vi "Main.vi"(9 "Graph Master":refnum<class "Graph Master.lvclass">=refnum, 10 "MIDA COM":refnum<visa-resource-name>="COM11", 11 "Module Admin":refnum<class "Delacor_lib_QMH_Module Admin.lvclass">) -> ()   [LabVIEW 2023, in "Drive.lvlib"]
doc: "This template is based off of the Queued Message Handler design pattern and the Queued Message Handler project template that ships with LabVIEW.\n\nThe main difference is that the queue is private to this module and communication between modules is performed via Broadcast and Request events.\n\nRequest events are wrapped in public API methods and are handled in the Event Handling Loop (EHL) of this VI. Any module can register for Broadcast events sent by this module. The EHL generates messages based on user interface actions.\n\nThe Message Handling Loop (MHL) processes messages generated by the EHL, or by other messages. The messages are string values, so new messages can be added easily to the Message Cases case structure in the MHL. Each message cluster can also provide an optional value for Message Data, which is a variant that can be converted to whatever message-specific data is required.\n_____\nBased on DQMH Project Template 6.1.0.94."
uses:
  Drive.lvlib
  <vilib>/Delacor/Delacor QMH/Libraries/Message Queue_class/Delacor_lib_QMH_Message Queue.lvclass
  Module Data--cluster.ctl
  <vilib>/Utility/miscctls.llb/LVPointTypeDef.ctl
  <vilib>/Utility/error.llb/Error Cluster From Error Code.vi
  <vilib>/ErrorRing/Error Ring.xnode
  <vilib>/Delacor/Delacor QMH/Libraries/Message Queue_class/Delacor_lib_QMH_Enqueue Message (Single).vi
  Stop Argument--cluster.ctl
  <vilib>/Delacor/Delacor QMH/Libraries/Module Admin_class/Delacor_lib_QMH_Module Admin.lvclass
  Kinco Drive/Kinco Type Class.ctl
  Kinco Drive/Drive_Status Argument--cluster.ctl
  <vilib>/ptbypt/NI_PtbyPt.lvlib
  <vilib>/NI/Modbus Library/API/Wrapper/API Main.lvlib
  <vilib>/NI/Modbus Library/API/Master/Modbus Master.lvclass
  Scheduler/Event Type.ctl
  Scheduler/Stop Argument--cluster.ctl
  Graph_data_collector/Stop event Type.ctl
  Scheduler/Events.ctl
  Scheduler/Init Type.ctl
  Pump_Data_Type.ctl
  Start_Pressure Argument--cluster.ctl
  Start_Mix Argument--cluster.ctl
  Calc_Type.ctl
  <vilib>/Utility/config.llb/NI_LVConfig.lvlib
  PVT_Drive_Type.ctl
  Save Type.ctl
  SubPanel Argument--cluster.ctl
  Rotation Control Type.ctl
  <vilib>/Kortex/Actor Planer/Actor Planer.lvlib
  <vilib>/ActorFramework/Message Enqueuer/Message Enqueuer.lvclass
  Graph Master/rqp_Create Graph.ctl
  KM20 Argument--cluster.ctl
  <vilib>/NI/Modbus Library/API/Wrapper/Create Serial Master.vi
  <vilib>/NI/Modbus Library/API/Wrapper/Create TCP Master.vi
  Mix Type.ctl
  Graph Master/Graph Master.lvclass
panel:
  out "MM PV":dbl(slide) caption="Положение PVT насоса" scale format="%#.2f"
  in  "Pop-Out Tool":bool
  out "P3":dbl caption="Датчик давления Р3" format="%.3f"
  out "P2":dbl caption="Датчик давления Р2" format="%.3f"
  in  "КМ20-40М":bool
  in  "KE":bool
  in  "K 6":bool
  in  "K 5":bool
  in  "K 4":bool
  in  "K 3":bool
  in  "K 2":bool
  in  "K 1":bool
  out "Pressure PV 2":dbl caption="Датчик давления Р4" format="%.3f"
  out "Pressure PV":dbl caption="Датчик давления Р5" format="%.3f"
  in  "TN 2":sgl=12.0 caption="TN" min=0 max=100 format="TN: %#.5f"
  in  "KP 2":sgl=750.0 caption="KP" min=0 max=10000 format="KP: %#.5f"
  in  "Насос":T1={"Mode"=1, "Pressure PV"=0.0, "Pressure SP"=0.0, "Flow PV"=0.0, "Flow SP"=0.0, "Volume PV"=0.0, "Volume SP"=0.0, "MM PV"=0.0, "Start"=FALSE, "Home"=FALSE} {"MM PV" scale format="%#.2f"; "Volume SP" min=0.0 max=1000.0 format="%.3f"; "Volume PV" format="%.3f"; "Flow SP" min=-300.0 max=300.0 format="%.3f"; "Flow PV" format="%.3f"; "Pressure SP" min=0.0 max=99.99 format="%.3f"; "Pressure PV" format="%.3f"; "Mode" items=["Давление"=1, "Расход"=2, "Объём"=3, "Извлечение"=4]}
  in  "Rotate":T2={"Mode"=1, "PV Angle"=0.0, "SP_Angle"=0.0, "Rotate Angle"=0.0, "Timeout"=0.0, "Start"=FALSE, "Home"=FALSE} caption="Поворот" {"Rotate Angle" format="%.1f"; "SP_Angle" format="%.1f"; "PV Angle" format="%.2f"; "Mode" items=["Поворот"=1, "Качание"=2]}
  out "P":dbl format="%.3f МПа"
  in  "TN":sgl=12.0 min=0 max=100 format="TN: %#.5f"
  in  "KP":sgl=750.0 min=0 max=10000 format="KP: %#.5f"
  in  "PVT":T1={"Mode"=1, "Pressure PV"=0.0, "Pressure SP"=0.0, "Flow PV"=0.0, "Flow SP"=0.0, "Volume PV"=0.0, "Volume SP"=0.0, "MM PV"=0.0, "Start"=FALSE, "Home"=FALSE} {"MM PV" scale format="%#.2f"; "Volume SP" min=0.0 max=1000.0 format="%.3f"; "Volume PV" format="%.3f"; "Flow SP" min=-300.0 max=300.0 format="%.3f"; "Flow PV" format="%.3f"; "Pressure SP" min=0.0 max=99.99 format="%.3f"; "Pressure PV" format="%.3f"; "Mode" items=["Давление"=1, "Расход"=2, "Объём"=3, "Извлечение"=4]}
  in  "MIX":T3 caption="Мешалка" {"Q" min=0.0 max=1000.0 format="%#.1f об/мин"}
  out "error out":errorcluster
  # "P2"
  # "P3"
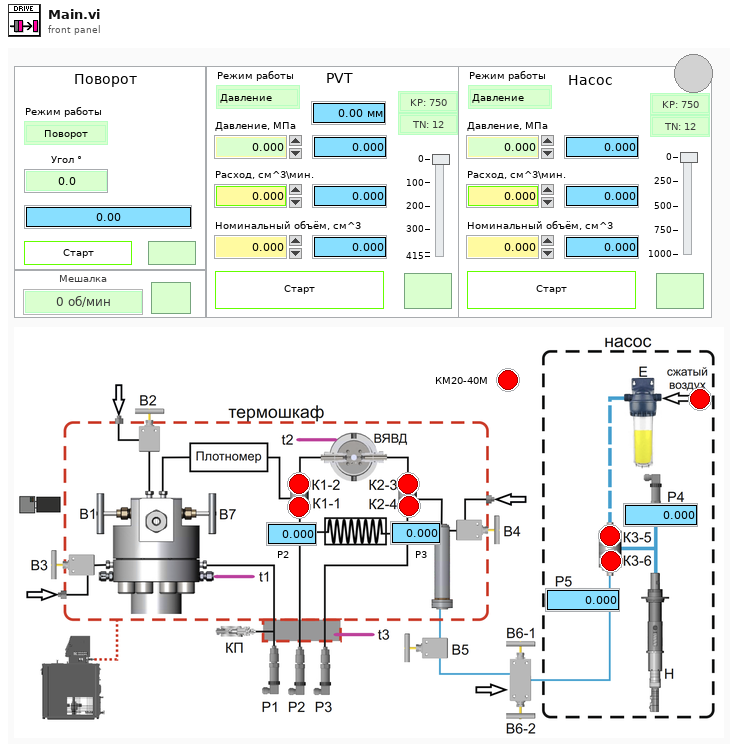
[diagram p1: front panel]
types:
  T1 = typedef "Drive.lvlib/PVT_Drive_Type.ctl" = cluster{"Mode":u16, "Pressure PV":dbl, "Pressure SP":dbl, "Flow PV":dbl, "Flow SP":dbl, "Volume PV":dbl, "Volume SP":dbl, "MM PV":dbl, "Start":bool, "Home":bool}
  T2 = typedef "Drive.lvlib/Rotation Control Type.ctl" = cluster{"Mode":u16, "PV Angle":dbl, "SP_Angle":dbl, "Rotate Angle":dbl, "Timeout":dbl, "Start":bool, "Home":bool}
  T3 = typedef "Drive.lvlib/Mix Type.ctl" = cluster{"Q":dbl, "on":bool}
  T4 = typedef "Kinco Drive.lvlib/Kinco Type Class.ctl" = enum16{"Position", "Speed"}
  T5 = typedef "Drive.lvlib/Request Events--cluster.ctl" = cluster{"Stop Module":refnum<user-event>, "Show Panel":refnum<user-event>, "Hide Panel":refnum<user-event>, "Get Module Execution Status":refnum<user-event>, "Show Diagram":refnum<user-event>, "Start_Pressure":refnum<user-event>, "Start_Mix":refnum<user-event>, "SubPanel":refnum<user-event>, "KM20":refnum<user-event>}
  T6 = typedef "Dispatcher.lvlib/Broadcast Events--cluster.ctl" = cluster{"Module Did Init":refnum<user-event>, "Status Updated":refnum<user-event>, "Error Reported":refnum<user-event>, "Module Did Stop":refnum<user-event>, "Update Module Execution Status":refnum<user-event>, "Emerg Stop Broad":refnum<user-event>}
  T7 = typedef "Settings Master.lvlib/Broadcast Events--cluster.ctl" = cluster{"Module Did Init":refnum<user-event>, "Status Updated":refnum<user-event>, "Error Reported":refnum<user-event>, "Module Did Stop":refnum<user-event>, "Update Module Execution Status":refnum<user-event>, "Settings":refnum<user-event>}
  T8 = typedef "Kinco Drive.lvlib/Broadcast Events--cluster.ctl" = cluster{"Module Did Init":refnum<user-event>, "Status Updated":refnum<user-event>, "Error Reported":refnum<user-event>, "Module Did Stop":refnum<user-event>, "Update Module Execution Status":refnum<user-event>, "Drive_Status":refnum<user-event>}
  T9 = typedef "Heat UI.lvlib/Broadcast Events--cluster.ctl" = cluster{"Module Did Init":refnum<user-event>, "Status Updated":refnum<user-event>, "Error Reported":refnum<user-event>, "Module Did Stop":refnum<user-event>, "Update Module Execution Status":refnum<user-event>, "T Data":refnum<user-event>, "Temp array":refnum<user-event>}
  T10 = typedef "Drive.lvlib/Module Data--cluster.ctl" = cluster{"Status":string, "Mix_ID":i32, "Rotate_ID":i32, "Rotate status":T11, "MB":refnum<class "Modbus Master.lvclass">, "Init":T12, "Temp array":dbl[], "Расчёты":T15, "Plan Enqueuer":refnum<class "Message Enqueuer.lvclass">, "mida":refnum<class "Modbus Master.lvclass">, "Subpanel Ref":refnum<vi>}
  T11 = typedef "Kinco Drive.lvlib/Drive_Status Argument--cluster.ctl" = cluster{"Module ID":i32, "Connection":bool, "is Home?":bool, "Position":dbl, "Done?":bool}
  T12 = typedef "Scheduler Lib.lvlib/Init Type.ctl" = cluster{"Message Queue in":refnum<class "Delacor_lib_QMH_Message Queue.lvclass">, "Events":T13}
  T13 = typedef "Scheduler Lib.lvlib/Events.ctl" = cluster{"Stop Module":T14, "Add event":refnum<user-event>}
  T14 = typedef "Scheduler Lib.lvlib/Stop event Type.ctl" = refnum<user-event>
  T15 = typedef "Drive.lvlib/Calc_Type.ctl" = cluster{"Vm0":dbl, "aa":dbl, "bb":dbl, "K0":dbl, "A":dbl, "B":dbl}
  T16 = enum32{"invalid lock state", "Not Locked", "Locked (No Password)", "Password-protected"}
  T17 = typedef "Drive.lvlib/Stop Argument--cluster.ctl" = cluster{"Origin":string, "Exit via Stop Module Req?":bool, "Wait for Module to stop?":bool}
  T18 = typedef "Graph Master.lvclass/rqp_Create Graph.ctl" = cluster{"Control ref":refnum<vi>}
  T19 = typedef "Drive.lvlib/Start_Pressure Argument--cluster.ctl" = cluster{"Pressure":dbl, "Start":bool}
  T20 = typedef "Drive.lvlib/Start_Mix Argument--cluster.ctl" = cluster{"RPM":dbl, "Start":bool}
  T21 = typedef "Drive.lvlib/SubPanel Argument--cluster.ctl" = cluster{"Sub Panel":refnum<vi>}
  T22 = typedef "Drive.lvlib/KM20 Argument--cluster.ctl" = cluster{"Обдув":bool}
  T23 = typedef "LVPointTypeDef.ctl" = cluster{"Horizontal":i16, "Vertical":i16}
  T24 = enum32{"Invalid", "Standard", "Closed", "Hidden", "Minimized", "Maximized"}
  T25 = typedef "Drive.lvlib/Pump_Data_Type.ctl" = cluster{"Pressure PV":dbl, "Flow PV":dbl, "Volume PV":dbl, "Position_MM":dbl, "Volume corrected":dbl, "mix rpm":dbl}
  T26 = enum8{"Enabled", "Disabled", "Disabled and Grayed Out"}
  T27 = typedef "Drive.lvlib/Save Type.ctl" = cluster{"Q mix":dbl, "Angle":dbl, "KP":sgl, "TN":sgl, "PVT":T1, "Rotate":T2, "Насос":T1, "KP 2":sgl, "TN 2":sgl}
  T28 = typedef "Heat UI.lvlib/Settings Type.ctl" = cluster{"KPтерм":dbl, "TNтерм":dbl, "KPниз":dbl, "TNниз":dbl, "COM ADC":refnum<visa-resource-name>, "COM Termex":refnum<visa-resource-name>, "KPдд":dbl, "TNдд":dbl, "Multiper":dbl}
  T29 = typedef "Menu.lvlib/Setts.ctl" = cluster{"IP adress":string}
  T30 = cluster{"Heat":T28, "Расчёты":T15, "Видеосистема":bool, "Anton Paar":T29, "MIDA COM":refnum<visa-resource-name>}
  T31 = typedef "NI_LVConfig.lvlib/Config Data RefNum.ctl" = refnum<k1>
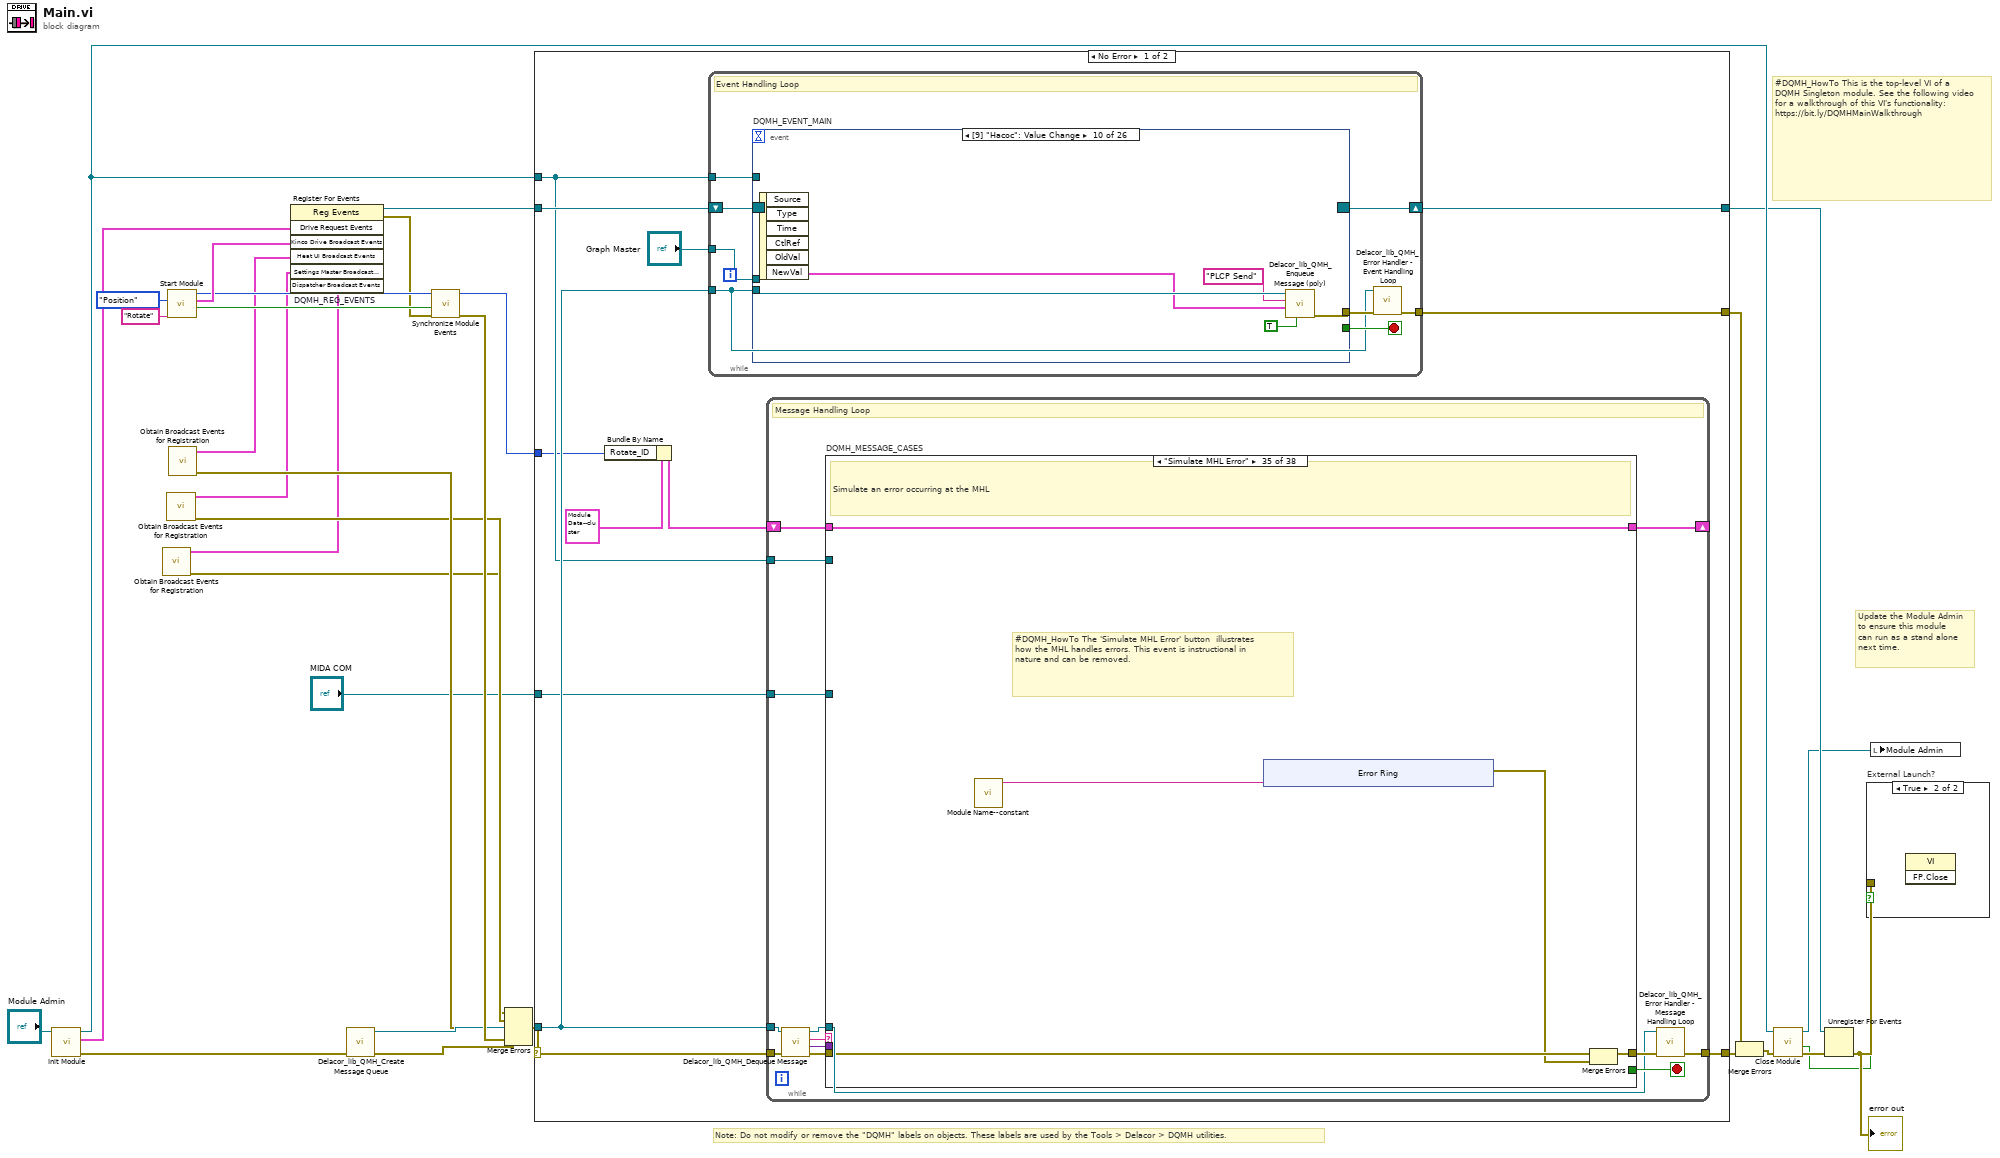
[diagram p0: block diagram]
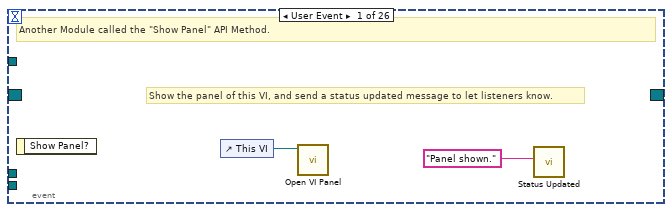
[diagram p3: hidden frame]
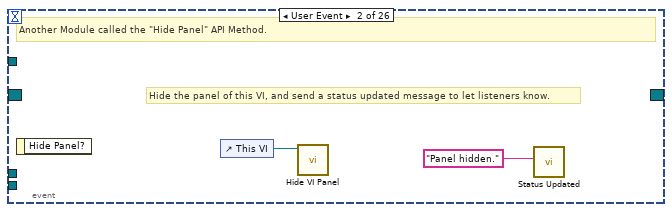
[diagram p4: hidden frame]
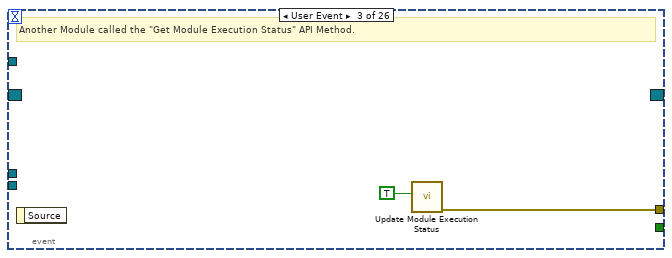
[diagram p5: hidden frame]
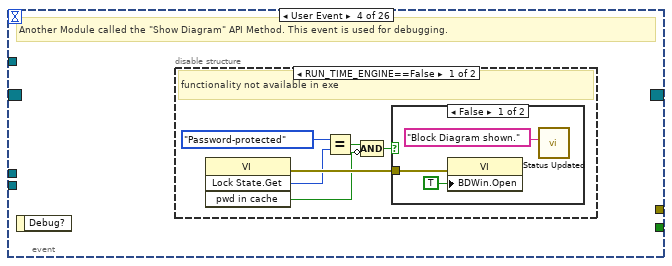
[diagram p6: hidden frame]
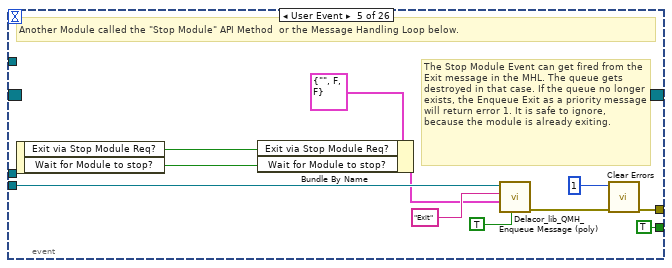
[diagram p9: hidden frame]
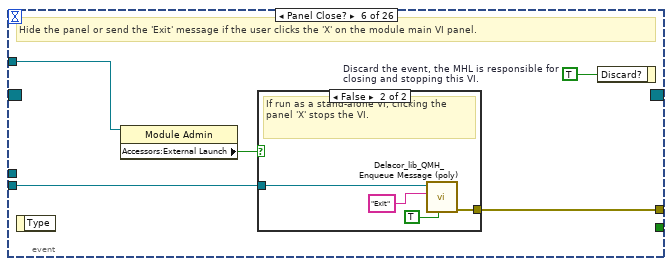
[diagram p10: hidden frame]
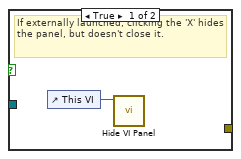
[diagram p11: hidden frame]
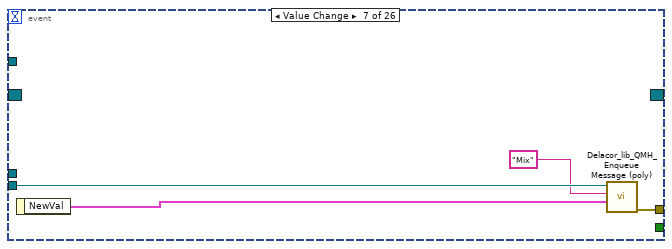
[diagram p12: hidden frame]
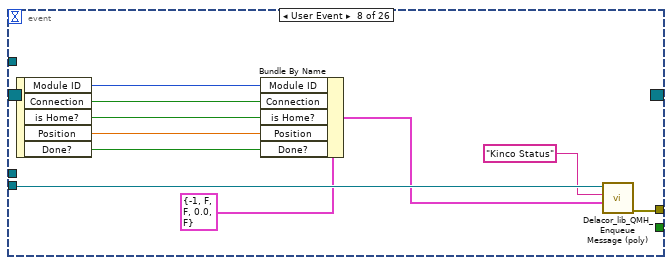
[diagram p13: hidden frame]
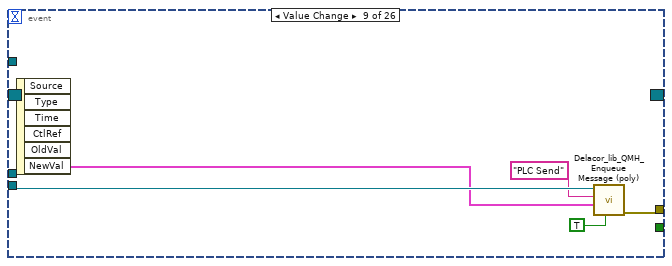
[diagram p14: hidden frame]
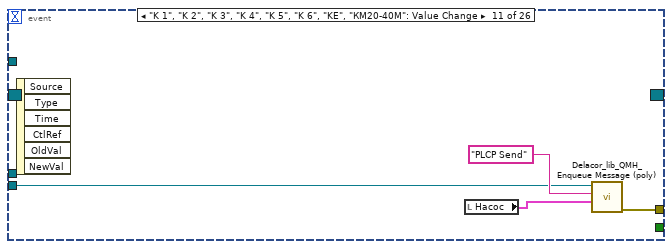
[diagram p15: hidden frame]
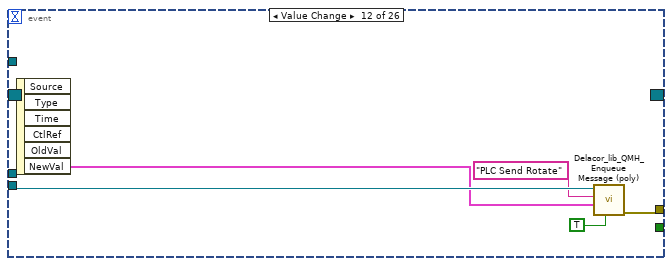
[diagram p16: hidden frame]
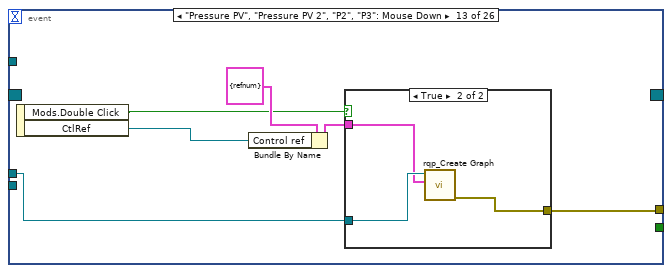
[diagram p17: hidden frame]
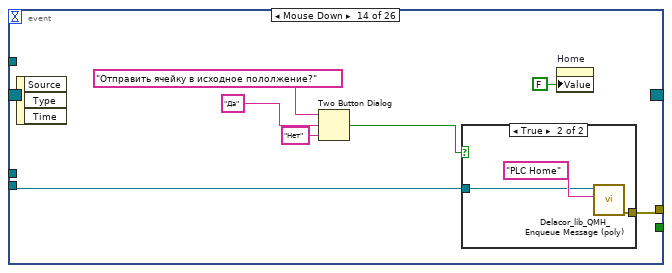
[diagram p19: hidden frame]
diagram:
  # "#DQMH_HowTo This is the top-level VI of a DQMH Singleton module. See the following video for a walkthrough of this VI's functionality: https://bit.ly/DQMHMainWalkthrough"
  # "Note: Do not modify or remove the \"DQMH\" labels on objects. These labels are used by the Tools > Delacor > DQMH utilities."
  # "Update the Module Admin to ensure this module can run as a stand alone next time."
  n1 = call "Init Module.vi"("Singleton Module Admin in"="Module Admin") -> ("error out"=w30:errorcluster, "Drive Request Events"=w8:T5, "Singleton Module Admin out"=w23:refnum<class "Delacor_lib_QMH_Module Admin.lvclass">)  [unwired: 8 in]
  n2 = call "Obtain Broadcast Events for Registration.vi"() -> ("error out"=w2:errorcluster, "Dispatcher Broadcast Events"=w3:T6)  [unwired: 9 in, 1 out]
  n3 = call "Obtain Broadcast Events for Registration.vi"() -> ("error out"=w4:errorcluster, "Settings Master Broadcast Events"=w5:T7)  [unwired: 9 in, 1 out]
  n4 = call "Start Module.vi"("File_name"="Rotate", "Kinco Type"=Kinco_Type_Class."Position") -> ("Wait for Event Sync?"=w16:bool, "Kinco Drive Broadcast Events"=w17:T8, "Module ID"=w15:i32)  [unwired: 6 in, 1 out]
  n5 = call "Obtain Broadcast Events for Registration.vi"() -> ("error out"=w6:errorcluster, "Heat UI Broadcast Events"=w7:T9)  [unwired: 9 in, 1 out]
  n6 = register-events "DQMH_REG_EVENTS"(w8, w17, w7, w5, w3) -> (reference out=w21:refnum<event-registration>, error out=w10:errorcluster)  [unwired: 2 in]
  n7 = call <vilib>:"Delacor_lib_QMH_Create Message Queue.vi"("error in"=w30) -> ("error out"=w25:errorcluster, "Message Queue"=w9:refnum<class "Delacor_lib_QMH_Message Queue.lvclass">)  [unwired: 9 in]
  n8 = call "Synchronize Module Events.vi"("error in"=w10, "Wait for Event Sync?"=w16, "Module ID in"=w15) -> ("error out"=w11:errorcluster, "Module ID out"=w12:i32)  [unwired: 7 in]
  n9 = Merge Errors(w2, w4, w6, w11, w25) -> (w24:errorcluster)
  n10 = case shown="No Error" w24 {
    selector: w24 -> [w41 w926]
    tunnel: [w43 w925] -> w31
    tunnel: [w40 w931] -> w22
    tunnel: w21 -> [w38 w931]
    tunnel: w9 -> [w37 w924]
    tunnel: [w42 _] -> w28
    tunnel: w23 -> [w36 w927]
    tunnel: w12 -> [w34 _]
    tunnel: "MIDA COM" -> [w33 _]
    frame No Error {
      n11 = Bundle By Name(cluster=T10 {"Status"="", "Mix_ID"=0, "Rotate_ID"=0, "Rotate status"={"Module ID"=0, "Connection"=FALSE, "is Home?"=FALSE, "Position"=0.0, "Done?"=FALSE}, "MB"=refnum, "Init"={"Message Queue in"=refnum, "Events"={"Stop Module"=refnum, "Add event"=refnum}}, "Temp array"=[], "Расчёты"={"Vm0"=8.0, "aa"=8.0, "bb"=8.0, "K0"=8.0, "A"=8.0, "B"=8.0}, "Plan Enqueuer"=refnum, "mida"=refnum, "Subpanel Ref"=refnum} ("Data Cluster"), "Rotate_ID"=w34) -> (w35:T10)
      n12 = while {
        tunnel: w37 -> [w45]
        shift-right: [w48] -> w40
        shift-left: w38 -> [w49]
        tunnel: [w50] -> w42
        tunnel: w36 -> [w46]
        tunnel: "Graph Master" -> [w44]
        stop <- w47 stop-if-true
        # "Event Handling Loop"
        n13 = event "DQMH_EVENT_MAIN" shown="[9] \"Насос\": Value Change" {
          selector: w49 -> [_ _ _ _ _ _ _ _ _ _ _ _ _ _ _ _ _ _ _ _ _ _ _ _ _ _]
          dyn-events: [_ _ _ _ _ _ _ _ _ _ _ _ _ _ _ _ _ _ _ _ _ _ _ _ _ _] -> w48
          timeout: _ -> [_ _ _ _ _ _ _ _ _ _ _ _ _ _ _ _ _ _ _ _ _ _ _ _ _ _]
          tunnel: [_ _ _ _ TRUE ("Discard?") _ _ _ _ _ _ _ _ _ _ _ _ _ _ _ _ _ _ _ _ _] -> w47
          tunnel: w45 -> [_ _ _ _ w73 w80 w90 w100 w105 w110 w113 w119 _ w135 w145 w155 w161 w164 w172 w179 w182 w187 w194 _ w205 w206]
          tunnel: [_ _ w57 _ w76 w82 w91 w101 w106 w111 w114 w120 w124 w136 w146 w156 w162 w165 w166 w173 w183 w188 w189 w197 w200 w207] -> w51
          tunnel: w46 -> [_ _ _ _ _ w79 _ _ _ _ _ _ _ _ _ _ _ _ _ _ _ _ _ _ _ _]
          tunnel: w44 -> [_ _ _ _ _ _ _ _ _ _ _ _ w121 _ _ _ _ _ _ _ _ _ _ _ _ _]
          event User Event {
            # "Show the panel of this VI, and send a status updated message to let listeners know."
            # "Another Module called the \"Show Panel\" API Method."
            n14 = event-data() -> ()  [unwired: 1 in, 1 out]
            n15 = control-ref of="This VI"() -> (w53:refnum<vi>)
            n16 = call "Open VI Panel.vi"("VI"=w53) -> ()  [unwired: 10 in, 1 out]
            n17 = call "Status Updated.vi"("Status"="Panel shown." ("format string")) -> ()  [unwired: 10 in, 1 out]
          }
          event User Event {
            # "Hide the panel of this VI, and send a status updated message to let listeners know."
            # "Another Module called the \"Hide Panel\" API Method."
            n18 = event-data() -> ()  [unwired: 1 in, 1 out]
            n19 = control-ref of="This VI"() -> (w55:refnum<vi>)
            n20 = call "Hide VI Panel.vi"("VI"=w55) -> ()  [unwired: 10 in, 1 out]
            n21 = call "Status Updated.vi"("Status"="Panel hidden." ("format string")) -> ()  [unwired: 10 in, 1 out]
          }
          event User Event {
            # "Another Module called the \"Get Module Execution Status\" API Method."
            n22 = event-data() -> ()  [unwired: 1 in, 1 out]
            n23 = call "Update Module Execution Status.vi"("Running?"=TRUE) -> ("error out"=w57:errorcluster)  [unwired: 10 in]
          }
          event User Event {
            # "Another Module called the \"Show Diagram\" API Method. This event is used for debugging."
            n24 = event-data() -> ()  [unwired: 1 in, 1 out]
            n25 = disable-structure shown="RUN_TIME_ENGINE==False" {
              frame condition #0 (active) {
                # "functionality not available in exe"
                n26 = invoke class="VI" method="Lock State.Get"() -> (error out=w63:errorcluster, "Get Lock State"=w62:T16, "pwd in cache"=w59:bool)  [unwired: 4 in, 1 out]
                n27 = Equal?(x=T16."Password-protected", y=w62) -> (x = y?=w60:bool)
                n28 = Compound Arithmetic op=AND(w60, invert w59) -> (w58:bool)
                n29 = case shown="False" w58 {
                  tunnel: w63 -> [w66 _]
                  frame False {
                    n30 = property class="VI"(error in=w66, "BDWin.Open"=TRUE ("Block Diagram Window:Open")) -> ()  [unwired: 1 in, 2 out]
                    n31 = call "Status Updated.vi"("Status"="Block Diagram shown." ("format string")) -> ()  [unwired: 10 in, 1 out]
                  }
                  frame True {
                    # "Password-protected VI, and the password is not in the cache. Do not show the diagram."
                  }
                }
              }
              frame condition #1 {
              }
            }
          }
          event User Event {
            # "The Stop Module Event can get fired from the Exit message in the MHL. The queue gets destroyed in that case. If the queue no longer exists, the Enqueue Exit as a priority message will return error 1. It is safe to ignore, because the module is already exiting."
            # "Another Module called the \"Stop Module\" API Method  or the Message Handling Loop below."
            n32 = event-data() -> ("Exit via Stop Module Req?"=w69:bool, "Wait for Module to stop?"=w68:bool)  [unwired: 1 in]
            n33 = Bundle By Name(cluster=T17 {"Origin"="", "Exit via Stop Module Req?"=FALSE, "Wait for Module to stop?"=FALSE} ("Stop Argument"), "Exit via Stop Module Req?"=w69, "Wait for Module to stop?"=w68) -> (w67:T17)
            n34 = call-poly <vilib>:"Delacor_lib_QMH_Enqueue Message (poly).vi"("Priority Message? (F)"=TRUE, "Message Data"=w67, "Message"="Exit", "Message Queue in"=w73) -> ("error out"=w77:errorcluster)  [unwired: 6 in, 1 out]
            n35 = call <vilib>:"Clear Errors.vi"("error in (no error)"=w77, "specific error code to clear (0: all)"=1) -> ("error out"=w76:errorcluster)  [unwired: 4 in, 1 out]
          }
          event Panel Close? {
            w81 = TRUE  # Discard the event, the MHL is responsible for closing and stopping this VI.
            # "Hide the panel or send the 'Exit' message if the user clicks the 'X' on the module main VI panel."
            n36 = event-data() -> ()  [unwired: 1 in, 1 out]
            n37 = property class="Module Admin"(reference=w79) -> ("Accessors:External Launch"=w78:bool)  [unwired: 1 in, 2 out]
            n38 = case shown="False" w78 {
              tunnel: w80 -> [_ w86]
              tunnel: [_ w87] -> w82
              frame True {
                # "If externally launched, clicking the 'X' hides the panel, but doesn't close it."
                n39 = control-ref of="This VI"() -> (w83:refnum<vi>)
                n40 = call "Hide VI Panel.vi"("VI"=w83) -> ()  [unwired: 10 in, 1 out]
              }
              frame False {
                # "If run as a stand-alone VI, clicking the panel 'X' stops the VI."
                n41 = call-poly <vilib>:"Delacor_lib_QMH_Enqueue Message (poly).vi"("Priority Message? (F)"=TRUE, "Message"="Exit", "Message Queue in"=w86) -> ("error out"=w87:errorcluster)  [unwired: 7 in, 1 out]
              }
            }
            n42 = event-data("Discard?"=w81) -> ()  [unwired: 1 in, 1 out]
          }
          event Value Change {
            n43 = event-data() -> ("NewVal"=w89:T3)  [unwired: 1 in]
            n44 = call-poly <vilib>:"Delacor_lib_QMH_Enqueue Message (poly).vi"("Message Data"=w89, "Message"="Mix", "Message Queue in"=w90) -> ("error out"=w91:errorcluster)  [unwired: 7 in, 1 out]
          }
          event User Event {
            n45 = event-data() -> ("Module ID"=w92:i32, "Connection"=w93:bool, "is Home?"=w94:bool, "Position"=w95:dbl, "Done?"=w96:bool)  [unwired: 1 in]
            n46 = Bundle By Name(cluster=T11 {"Module ID"=-1, "Connection"=FALSE, "is Home?"=FALSE, "Position"=0.0, "Done?"=FALSE} ("Drive_Status Argument"), "Module ID"=w92, "Connection"=w93, "is Home?"=w94, "Position"=w95, "Done?"=w96) -> (w97:T11)
            n47 = call-poly <vilib>:"Delacor_lib_QMH_Enqueue Message (poly).vi"("Message Data"=w97, "Message"="Kinco Status", "Message Queue in"=w100) -> ("error out"=w101:errorcluster)  [unwired: 7 in, 1 out]
          }
          event Value Change {
            n48 = event-data() -> ("NewVal"=w104:T1)  [unwired: 1 in, 5 out]
            n49 = call-poly <vilib>:"Delacor_lib_QMH_Enqueue Message (poly).vi"("Priority Message? (F)"=TRUE, "Message Data"=w104, "Message"="PLC Send", "Message Queue in"=w105) -> ("error out"=w106:errorcluster)  [unwired: 6 in, 1 out]
          }
          event Value Change {
            n50 = event-data() -> ("NewVal"=w109:T1)  [unwired: 1 in, 5 out]
            n51 = call-poly <vilib>:"Delacor_lib_QMH_Enqueue Message (poly).vi"("Priority Message? (F)"=TRUE, "Message Data"=w109, "Message"="PLCP Send", "Message Queue in"=w110) -> ("error out"=w111:errorcluster)  [unwired: 6 in, 1 out]
          }
          event "K 1", "K 2", "K 3", "K 4", "K 5", "K 6", "KE", "КМ20-40М": Value Change {
            n52 = event-data() -> ()  [unwired: 1 in, 6 out]
            n53 = local read "Насос"() -> (w112:T1)
            n54 = call-poly <vilib>:"Delacor_lib_QMH_Enqueue Message (poly).vi"("Message Data"=w112, "Message"="PLCP Send", "Message Queue in"=w113) -> ("error out"=w114:errorcluster)  [unwired: 7 in, 1 out]
          }
          event Value Change {
            n55 = event-data() -> ("NewVal"=w118:T2)  [unwired: 1 in, 5 out]
            n56 = call-poly <vilib>:"Delacor_lib_QMH_Enqueue Message (poly).vi"("Priority Message? (F)"=TRUE, "Message Data"=w118, "Message"="PLC Send Rotate", "Message Queue in"=w119) -> ("error out"=w120:errorcluster)  [unwired: 6 in, 1 out]
          }
          event "Pressure PV", "Pressure PV 2", "P2", "P3": Mouse Down {
            n57 = event-data() -> ("Mods.Double Click"=w123:bool, "CtlRef"=w122:refnum<vi>)  [unwired: 1 in]
            n58 = Bundle By Name(cluster=T18 {"Control ref"=refnum} ("Data in"), "Control ref"=w122) -> (w125:T18)
            n59 = case shown="True" w123 {
              tunnel: w121 -> [_ w129]
              tunnel: [_ w128] -> w124
              tunnel: w125 -> [_ w127]
              frame False {
              }
              frame True {
                n60 = call "rqp_Create Graph.vi"("Data in"=w127, "Graph Master in"=w129) -> ("error out"=w128:errorcluster)  [unwired: 7 in, 2 out]
              }
            }
          }
          event Mouse Down {
            n61 = event-data() -> ()  [unwired: 1 in, 3 out]
            n62 = Two Button Dialog(message="Отправить ячейку в исходное пололжение?", 1:"Нет" ("F button name (\"Cancel\")"), 2:"Да" ("T button name (\"OK\")")) -> (T button?=w130:bool)
            n63 = case shown="True" w130 {
              tunnel: [_ w139] -> w136
              tunnel: w135 -> [_ w137]
              frame False {
              }
              frame True {
                n64 = call-poly <vilib>:"Delacor_lib_QMH_Enqueue Message (poly).vi"("Message"="PLC Home", "Message Queue in"=w137) -> ("error out"=w139:errorcluster)  [unwired: 8 in, 1 out]
              }
            }
            n65 = property on="Home" class="Bool (strict)"("Value"=FALSE) -> ()  [unwired: 2 in, 2 out]
          }
          event Mouse Down {
            n66 = event-data() -> ()  [unwired: 1 in, 3 out]
            n67 = Two Button Dialog(message="Повернуть насос в исходное пололжение?", 1:"Нет" ("F button name (\"Cancel\")"), 2:"Да" ("T button name (\"OK\")")) -> (T button?=w140:bool)
            n68 = case shown="True" w140 {
              tunnel: [_ w149] -> w146
              tunnel: w145 -> [_ w147]
              frame False {
              }
              frame True {
                n69 = call-poly <vilib>:"Delacor_lib_QMH_Enqueue Message (poly).vi"("Message"="PLCP Home", "Message Queue in"=w147) -> ("error out"=w149:errorcluster)  [unwired: 8 in, 1 out]
              }
            }
            n70 = property on="Home" class="Bool (strict)"("Value"=FALSE) -> ()  [unwired: 2 in, 2 out]
          }
          event Mouse Down {
            n71 = event-data() -> ()  [unwired: 1 in, 3 out]
            n72 = Two Button Dialog(message="Повернуть ячейку в исходное пололжение?", 1:"Нет" ("F button name (\"Cancel\")"), 2:"Да" ("T button name (\"OK\")")) -> (T button?=w153:bool)
            n73 = case shown="True" w153 {
              tunnel: [_ w159] -> w156
              tunnel: w155 -> [_ w157]
              frame False {
              }
              frame True {
                n74 = call-poly <vilib>:"Delacor_lib_QMH_Enqueue Message (poly).vi"("Message"="PLC Rotate Home", "Message Queue in"=w157) -> ("error out"=w159:errorcluster)  [unwired: 8 in, 1 out]
              }
            }
            n75 = property on="Home" class="Bool (strict)"("Value"=FALSE) -> ()  [unwired: 2 in, 2 out]
          }
          event "KP", "TN": Value Change {
            n76 = event-data() -> ()  [unwired: 1 in, 6 out]
            n77 = call-poly <vilib>:"Delacor_lib_QMH_Enqueue Message (poly).vi"("Message"="Write PID", "Message Queue in"=w161) -> ("error out"=w162:errorcluster)  [unwired: 8 in, 1 out]
          }
          event "KP 2", "TN 2": Value Change {
            n78 = event-data() -> ()  [unwired: 1 in, 6 out]
            n79 = call-poly <vilib>:"Delacor_lib_QMH_Enqueue Message (poly).vi"("Message"="Write PIDP", "Message Queue in"=w164) -> ("error out"=w165:errorcluster)  [unwired: 8 in, 1 out]
          }
          event User Event {
            # "Another Module called the \"Start_Pressure\" API Method."
            n80 = event-data() -> ("Pressure"=w168:dbl, "Start"=w167:bool)  [unwired: 1 in]
            n81 = Bundle(cluster=T19 {"Pressure"=0.0, "Start"=FALSE} ("Start_Pressure Argument"), "Pressure"=w168, "Start"=w167) -> (w169:T19)
            n82 = call-poly <vilib>:"Delacor_lib_QMH_Enqueue Message (poly).vi"("Message Data"=w169, "Message"="Start_Pressure", "Message Queue in"=w172) -> ("error out"=w166:errorcluster)  [unwired: 7 in, 1 out]
          }
          event User Event {
            # "Another Module called the \"Start_Mix\" API Method."
            n83 = event-data() -> ("RPM"=w175:dbl, "Start"=w174:bool)  [unwired: 1 in]
            n84 = Bundle(cluster=T20 {"RPM"=0.0, "Start"=FALSE} ("Start_Mix Argument"), "RPM"=w175, "Start"=w174) -> (w176:T20)
            n85 = call-poly <vilib>:"Delacor_lib_QMH_Enqueue Message (poly).vi"("Message Data"=w176, "Message"="Start_Mix", "Message Queue in"=w179) -> ("error out"=w173:errorcluster)  [unwired: 7 in, 1 out]
          }
          event User Event {
            n86 = event-data() -> ("Temp array"=w181:dbl[])  [unwired: 1 in]
            n87 = call-poly <vilib>:"Delacor_lib_QMH_Enqueue Message (poly).vi"("Message Data"=w181, "Message"="Temp Data", "Message Queue in"=w182) -> ("error out"=w183:errorcluster)  [unwired: 7 in, 1 out]
          }
          event User Event {
            n88 = event-data() -> ("Main"=w186:T30)  [unwired: 1 in]
            n89 = Unbundle By Name(w186) -> ("Расчёты"=w185:T15)
            n90 = call-poly <vilib>:"Delacor_lib_QMH_Enqueue Message (poly).vi"("Message Data"=w185, "Message"="Setts", "Message Queue in"=w187) -> ("error out"=w188:errorcluster)  [unwired: 7 in, 1 out]
          }
          event User Event {
            # "Another Module called the \"SubPanel\" API Method."
            n91 = event-data() -> ("Sub Panel"=w190:refnum<vi>)  [unwired: 1 in]
            n92 = Bundle(cluster=T21 {"Sub Panel"=refnum} ("SubPanel Argument"), "Sub Panel"=w190) -> (w191:T21)
            n93 = call-poly <vilib>:"Delacor_lib_QMH_Enqueue Message (poly).vi"("Message Data"=w191, "Message"="SubPanel", "Message Queue in"=w194) -> ("error out"=w189:errorcluster)  [unwired: 7 in, 1 out]
          }
          event User Event {
            w196 = FALSE ("Value (Signaling)")
            n94 = event-data() -> ()  [unwired: 1 in, 1 out]
            n95 = property on="Start" class="Bool (strict)"("Val(Sgnl)"=w196) -> (error out=w199:errorcluster)  [unwired: 2 in, 1 out]
            n96 = property on="on" class="Bool (strict)"("Val(Sgnl)"=w196) -> (error out=w198:errorcluster)  [unwired: 2 in, 1 out]
            n97 = property on="Start" class="Bool (strict)"("Val(Sgnl)"=w196) -> (error out=w195:errorcluster)  [unwired: 2 in, 1 out]
            n98 = Merge Errors(w195, w198, w199) -> (w197:errorcluster)
          }
          event User Event {
            # "Another Module called the \"KM20\" API Method."
            n99 = event-data() -> ("Обдув"=w201:bool)  [unwired: 1 in]
            n100 = Bundle(cluster=T22 {"Обдув"=FALSE} ("KM20 Argument"), "Обдув"=w201) -> (w202:T22)
            n101 = call-poly <vilib>:"Delacor_lib_QMH_Enqueue Message (poly).vi"("Message Data"=w202, "Message"="KM20", "Message Queue in"=w205) -> ("error out"=w200:errorcluster)  [unwired: 7 in, 1 out]
          }
          event "Pop-Out Tool": Value Change {
            n102 = event-data() -> ()  [unwired: 1 in, 1 out]
            n103 = call-poly <vilib>:"Delacor_lib_QMH_Enqueue Message (poly).vi"("Message"="Window", "Message Queue in"=w206) -> ("error out"=w207:errorcluster)  [unwired: 8 in, 1 out]
          }
        }
        n104 = call-dynamic "Delacor_lib_QMH_Error Handler - Event Handling Loop.vi"("error in"=w51, "Message Queue in"=w45) -> ("dup error in"=w50:errorcluster)  [unwired: 8 in, 1 out]
      }
      n105 = while {
        tunnel: w37 -> [w212]
        shift-right: [w216] -> _
        shift-left: w35 -> [w217]
        tunnel: w41 -> [w220]
        tunnel: [w218] -> w43
        tunnel: w36 -> [w210]
        tunnel: w33 -> [w209]
        stop <- w215 stop-if-true
        # "Message Handling Loop"
        n106 = call-dynamic "Delacor_lib_QMH_Dequeue Message.vi"("error in"=w220, "Message Queue in"=w212) -> ("error out"=w219:errorcluster, "Message Data"=w213:variant, "Message"=w214:string, "Message Queue out"=w211:refnum<class "Delacor_lib_QMH_Message Queue.lvclass">)  [unwired: 6 in]
        n107 = case "DQMH_MESSAGE_CASES" shown="\"Simulate MHL Error\"" w214 {
          selector: w214 -> [_ _ _ _ _ _ _ _ _ _ _ _ _ _ _ _ _ _ _ _ _ _ _ _ _ _ _ _ _ _ _ _ _ _ _ _ _ w911]
          tunnel: w211 -> [w227 _ _ _ _ _ _ _ _ _ _ w378 _ _ _ _ w475 _ _ _ w540 w604 w640 _ w682 w713 w740 _ _ _ _ _ w810 _ _ w853 w903 _]
          tunnel: w219 -> [w253 w256 w269 w281 w292 w301 w304 w313 w334 w361 w377 w386 w395 w407 w433 w455 w493 w506 _ w528 w557 w614 w651 w678 w694 w724 w744 _ _ w777 w798 w806 w821 w838 w843 w860 w909 w913]
          tunnel: [w236 w256 w258 w271 w286 w294 w303 w312 w333 w360 w376 w385 w394 w409 w435 w457 w492 w508 w522 w530 w556 w613 w650 w679 w695 w725 w745 w759 w773 w783 w803 w808 w822 w838 w842 w856 w906 w914] -> w221
          tunnel: w217 -> [w244 w255 w268 w280 w291 w300 w302 w311 w332 w359 w367 w384 w391 w408 w434 w456 w491 w507 w521 w529 w532 w605 w644 w670 w690 w721 w734 w758 w772 w782 w802 w807 w818 w837 w840 w855 w890 w912]
          tunnel: [w243 w255 w268 w280 w283 w300 w302 w311 w327 w344 w370 w384 w391 w408 w434 w456 w491 w503 w520 w524 w539 w603 w647 w670 w685 w716 w734 w754 w768 w779 w800 w807 w816 w837 w840 w855 w890 w912] -> w216
          tunnel: [_ _ _ _ _ _ _ _ _ _ _ _ _ _ _ _ _ _ _ _ _ _ _ _ _ _ _ _ _ _ _ _ _ _ _ _ w902 _] -> w215
          tunnel: w213 -> [_ _ w266 w278 w289 w298 _ _ _ _ _ _ _ w405 w431 w453 _ w505 _ w527 _ _ _ w677 w693 w723 w743 _ _ _ _ _ w820 _ _ w854 w901 _]
          tunnel: w210 -> [w245 _ _ _ _ _ _ _ _ _ _ _ _ _ _ _ _ _ _ _ _ _ _ _ _ _ _ _ _ _ _ _ _ _ _ w852 w896 _]
          tunnel: w209 -> [_ _ _ _ _ _ _ _ _ _ w362 _ _ _ _ _ _ _ _ _ _ _ _ _ _ _ _ _ _ _ _ _ _ _ _ _ _ _]
          frame "Initialize" {
            # "Initialize - Any operation that needs to be done before the module can receive messages. Synchronize Caller Events.vi will inform Start Module.vi that the module has launched and is ready to receive messages. Module Did Init.vi will broadcast that the module initialized."
            n108 = call "Synchronize Caller Events.vi"("error in (no error)"=w253, "Singleton Module Admin in"=w245) -> ("error out"=w252:errorcluster, "Singleton Module Admin out"=w240:refnum<class "Delacor_lib_QMH_Module Admin.lvclass">)  [unwired: 8 in]
            n109 = property class="Module Admin"(reference=w240) -> ("Accessors:External Launch"=w249:bool)  [unwired: 1 in, 2 out]
            n110 = property on="Pane" class="Pane"("Origin"=T23 {"Horizontal"=0, "Vertical"=0}) -> ()  [unwired: 2 in, 2 out]
            n111 = call-poly <vilib>:"Delacor_lib_QMH_Enqueue Message (poly).vi"("Message"="Load param", "Message Queue in"=w227) -> ("error out"=w230:errorcluster, "Message Queue out"=w228:refnum<class "Delacor_lib_QMH_Message Queue.lvclass">)  [unwired: 8 in]
            n112 = Select(t=T24."Hidden" ("State"), s=w249, f=T24."Standard" ("State")) -> (s? t:f=w246:T24)
            n113 = call-poly <vilib>:"Delacor_lib_QMH_Enqueue Message (poly).vi"("error in"=w230, "Message"="PLC Connect", "Message Queue in"=w228) -> ("error out"=w229:errorcluster, "Message Queue out"=w235:refnum<class "Delacor_lib_QMH_Message Queue.lvclass">)  [unwired: 7 in]
            n114 = call-poly <vilib>:"Delacor_lib_QMH_Enqueue Message (poly).vi"("error in"=w229, "Message"="Read Setts", "Message Queue in"=w235) -> ("error out"=w225:errorcluster, "Message Queue out"=w226:refnum<class "Delacor_lib_QMH_Message Queue.lvclass">)  [unwired: 7 in]
            n115 = call-poly <vilib>:"Delacor_lib_QMH_Enqueue Message (poly).vi"("error in"=w225, "Message"="MIDA open", "Message Queue in"=w226) -> ("error out"=w223:errorcluster, "Message Queue out"=w224:refnum<class "Delacor_lib_QMH_Message Queue.lvclass">)  [unwired: 7 in]
            n116 = call <vilib>:"Start.vi"("DQMH Queue"=w224) -> ("error out"=w231:errorcluster, "Plan Enqueuer"=w232:refnum<class "Message Enqueuer.lvclass">)  [unwired: 9 in]
            n117 = property class="VI"("Front Panel.Title"="Управление движениями" ("Front Panel Window:Title")) -> (reference out=w250:refnum<vi>, error out=w254:errorcluster)  [unwired: 2 in]
            n118 = call "Module Name--constant.vi"() -> ("Module Name"=w241:string)  [unwired: 11 in]
            n119 = invoke class="VI" method="FP.Open"(reference=w250, error in=w254, "State"=w246) -> ()  [unwired: 2 in, 5 out]
            n120 = Bundle By Name(cluster=w244, "Plan Enqueuer"=w232) -> (w243:T10)
            n121 = call "Module Did Init.vi"("error in (no error)"=w252, "Initialized?"=TRUE, "Origin"=w241) -> ("error out"=w251:errorcluster)  [unwired: 8 in]
            n122 = Merge Errors(w231, w223, w251) -> (w236:errorcluster)
          }
          frame "---Module Specific---" {
            # "Separator -- The following cases handle messages specific to this Module."
          }
          frame "Start_Pressure" {
            n123 = Variant To Data(error in=w269, type=T19 {"Pressure"=0.0, "Start"=FALSE} ("Start_Pressure Argument"), Variant=w266) -> (data=w264:T19, error out=w267:errorcluster)
            n124 = Unbundle By Name(w264) -> ("Pressure"=w261:dbl, "Start"=w260:bool)
            n125 = local read "PVT"() -> (w263:T1)
            n126 = Bundle By Name(cluster=w263, "Mode"=u16 1, "Pressure SP"=w261, "Start"=w260) -> (w259:T1)
            n127 = property on="PVT" class="Clust (strict)"("Val(Sgnl)"=w259) -> (error out=w257:errorcluster)  [unwired: 2 in, 1 out]
            n128 = Merge Errors(w257, w267) -> (w258:errorcluster)
          }
          frame "Start_Mix" {
            n129 = Variant To Data(error in=w281, type=T20 {"RPM"=0.0, "Start"=FALSE} ("Start_Mix Argument"), Variant=w278) -> (data=w276:T20, error out=w279:errorcluster)
            n130 = Unbundle By Name(w276) -> ("RPM"=w274:dbl, "Start"=w273:bool)
            n131 = local read "MIX"() -> (w275:T3)
            n132 = Bundle By Name(cluster=w275, "Q"=w274, "on"=w273) -> (w272:T3)
            n133 = property on="MIX" class="Clust (strict)"("Val(Sgnl)"=w272) -> (error out=w270:errorcluster)  [unwired: 2 in, 1 out]
            n134 = Merge Errors(w270, w279) -> (w271:errorcluster)
          }
          frame "SubPanel" {
            n135 = Variant To Data(error in=w292, type=T21 {"Sub Panel"=refnum} ("SubPanel Argument"), Variant=w289) -> (data=w287:T21, error out=w290:errorcluster)
            n136 = Unbundle By Name(w287) -> ("Sub Panel"=w282:refnum<vi>)
            n137 = control-ref of="This VI"() -> (w284:refnum<vi>)
            n138 = Bundle By Name(cluster=w291, "Subpanel Ref"=w282) -> (w283:T10)
            n139 = call "Insert SubPanel.vi"("VI Ref"=w284, "Subpanel Ref"=w282) -> ("error out"=w285:errorcluster)  [unwired: 9 in]
            n140 = Merge Errors(w285, w290) -> (w286:errorcluster)
          }
          frame "KM20" {
            n141 = Variant To Data(error in=w301, type=T22 {"Обдув"=FALSE} ("KM20 Argument"), Variant=w298) -> (data=w296:T22, error out=w299:errorcluster)
            n142 = Unbundle By Name(w296) -> ("Обдув"=w295:bool)
            n143 = property on="КМ20-40М" class="Bool (strict)"("Val(Sgnl)"=w295) -> (error out=w293:errorcluster)  [unwired: 2 in, 1 out]
            n144 = Merge Errors(w293, w299) -> (w294:errorcluster)
          }
          frame "---Copy This Frame---" {
            # "Duplicate this frame when creating new messages.  Change this comment in the duplicated frame to describe this message."
            n145 = Merge Errors(w304) -> (w303:errorcluster)
          }
          frame "Window" {
            # "Duplicate this frame when creating new messages.  Change this comment in the duplicated frame to describe this message."
            n146 = Unbundle By Name(w311) -> ("Subpanel Ref"=w306:refnum<vi>)
            n147 = control-ref of="This VI"() -> (w309:refnum<vi>)
            n148 = invoke class="SubPnl" method="Remove VI"(reference=w306) -> (error out=w307:errorcluster)  [unwired: 2 in, 2 out]
            n149 = invoke class="VI" method="FP.Close"(reference=w309, error in=w307) -> (reference out=w310:refnum<vi>)  [unwired: 1 in, 2 out]
            n150 = invoke class="VI" method="FP.Open"(reference=w310, "State"=T24."Standard") -> (error out=w305:errorcluster)  [unwired: 3 in, 4 out]
            n151 = Merge Errors(w305, w313) -> (w312:errorcluster)
          }
          frame "ReadDO" {
            # "Duplicate this frame when creating new messages.  Change this comment in the duplicated frame to describe this message."
            n152 = Unbundle By Name(w332) -> ("MB"=w331:refnum<class "Modbus Master.lvclass">)
            n153 = call-dynamic "Read Holding Registers.vi"("number of inputs"=u16 1, "starting address"=u16 50, "Modbus master in"=w331) -> ("error out"=w328:errorcluster, "register values"=w325:u16[], "Modbus master out"=w326:refnum<class "Modbus Master.lvclass">)  [unwired: 6 in]
            n154 = Index Array(array=w325) -> (element=w324:u16)  [unwired: 1 in]
            n155 = Number To Boolean Array(number=w324) -> (Boolean array=w323:bool[])
            n156 = Bundle By Name(cluster=w332, "MB"=w326) -> (w327:T10)
            n157 = Index Array(array=w323, index #1=8 ("index")) -> (element #1=w321:bool, element #2=w320:bool, element #3=w319:bool, element #4=w318:bool, element #5=w317:bool, element #6=w316:bool, element #7=w315:bool, element #8=w314:bool)  [unwired: 7 in]
            n158 = local write "K 1"(w321) -> ()
            n159 = local write "K 2"(w320) -> ()
            n160 = local write "K 3"(w319) -> ()
            n161 = local write "K 4"(w318) -> ()
            n162 = local write "K 5"(w317) -> ()
            n163 = local write "K 6"(w316) -> ()
            n164 = local write "KE"(w315) -> ()
            n165 = local write "КМ20-40М"(w314) -> ()
            n166 = Merge Errors(w328, w334) -> (w333:errorcluster)
          }
          frame "MIDA read" {
            # "Duplicate this frame when creating new messages.  Change this comment in the duplicated frame to describe this message."
            n167 = Unbundle By Name(w359) -> ("mida"=w358:refnum<class "Modbus Master.lvclass">)
            n168 = call <vilib>:"Set Unit ID.vi"("unit ID"=u8 1, "Modbus master in"=w358) -> ("error out"=w356:errorcluster, "Modbus master out"=w355:refnum<class "Modbus Master.lvclass">)  [unwired: 8 in]
            n169 = call-dynamic "Read Input Registers.vi"("error in"=w356, "number of inputs"=u16 2, "starting address"=u16 2, "Modbus master in"=w355) -> ("error out"=w346:errorcluster, "register values"=w342:u16[], "Modbus master out"=w347:refnum<class "Modbus Master.lvclass">)  [unwired: 5 in]
            n170 = Index Array(array=w342) -> (element #1=w341:u16, element #2=w340:u16)  [unwired: 2 in]
            n171 = call "WORD_To_Float.vi"("second_Word"=w340, "first_Word"=w341) -> ("output_Float"=→"P3":sgl)  [unwired: 9 in]
            n172 = call <vilib>:"Set Unit ID.vi"("error in"=w346, "unit ID"=u8 2, "Modbus master in"=w347) -> ("error out"=w351:errorcluster, "Modbus master out"=w350:refnum<class "Modbus Master.lvclass">)  [unwired: 7 in]
            n173 = call-dynamic "Read Input Registers.vi"("error in"=w351, "number of inputs"=u16 2, "starting address"=u16 2, "Modbus master in"=w350) -> ("error out"=w345:errorcluster, "register values"=w337:u16[], "Modbus master out"=w343:refnum<class "Modbus Master.lvclass">)  [unwired: 5 in]
            n174 = Index Array(array=w337) -> (element #1=w338:u16, element #2=w339:u16)  [unwired: 2 in]
            n175 = call "WORD_To_Float.vi"("second_Word"=w339, "first_Word"=w338) -> ("output_Float"=→"P2":sgl)  [unwired: 9 in]
            n176 = Bundle By Name(cluster=w359, "mida"=w343) -> (w344:T10)
            n177 = Merge Errors(w345, w361) -> (w360:errorcluster)
          }
          frame "MIDA open" {
            w373 = u16 2 items=["None", "Odd", "Even", "Mark", "Space"] ("parity (even)")
            w375 = u16 0 items=["None", "XON/XOFF", "RTS/CTS", "XON/XOFF & RTS/CTS", "DTR/DSR", "XON/XOFF & DTR/DSR"] ("flow control (none)")
            # "Duplicate this frame when creating new messages.  Change this comment in the duplicated frame to describe this message."
            n178 = Unbundle By Name(w367) -> ("Plan Enqueuer"=w366:refnum<class "Message Enqueuer.lvclass">)
            n179 = call-poly <vilib>:"Create Modbus Instance.vi"("flow control (none)"=w375, "serial type"=enum16{"RTU", "ASCII"}."RTU", "parity (even)"=w373, "unit ID"=u8 1, "baud rate"=u32 19200, "VISA resource name"=w362) -> ("error out"=w368:errorcluster, "serial master instance"=w369:refnum<class "Modbus Master.lvclass">)  [unwired: 4 in]
            n180 = Bundle By Name(cluster=w367, "mida"=w369) -> (w370:T10)
            n181 = call <vilib>:"Add Event.vi"("Continius? (F)"=TRUE, "Action"="MIDA read", "Plan Enqueuer"=w366) -> ("error out"=w364:errorcluster)  [unwired: 6 in, 2 out]
            n182 = Merge Errors(w364, w368, w377) -> (w376:errorcluster)
          }
          frame "RStop" {
            # "Duplicate this frame when creating new messages.  Change this comment in the duplicated frame to describe this message."
            n183 = local read "Rotate"() -> (w381:T2)
            n184 = Bundle By Name(cluster=w381, "Start"=FALSE) -> (w379:T2)
            n185 = local write "Rotate"(w379) -> ()
            n186 = call-poly <vilib>:"Delacor_lib_QMH_Enqueue Message (poly).vi"("Message Data"=w379, "Message"="Update UI Rotate", "Message Queue in"=w378) -> ("error out"=w382:errorcluster)  [unwired: 7 in, 1 out]
            n187 = Merge Errors(w382, w386) -> (w385:errorcluster)
          }
          frame "PLC Read Rotate" {
            # "Duplicate this frame when creating new messages.  Change this comment in the duplicated frame to describe this message."
            n188 = Unbundle By Name(w391) -> ("Rotate status.Position"=w389:dbl)  [unwired: 3 out]
            n189 = local read "Rotate"() -> (w392:T2)
            n190 = Divide(x=w389, y=18204.444444444445) -> (x/y=w388:dbl)
            n191 = Bundle By Name(cluster=w392, "PV Angle"=w388) -> (w390:T2)
            n192 = local write "Rotate"(w390) -> ()
            n193 = call "Rotate Data.vi"("Rotate"=w390) -> ("error out"=w393:errorcluster)  [unwired: 10 in]
            n194 = Merge Errors(w393, w395) -> (w394:errorcluster)
          }
          frame "Update UI" {
            # "Duplicate this frame when creating new messages.  Change this comment in the duplicated frame to describe this message."
            n195 = Variant To Data(error in=w407, type=T1 {"Mode"=1, "Pressure PV"=0.0, "Pressure SP"=0.0, "Flow PV"=0.0, "Flow SP"=0.0, "Volume PV"=0.0, "Volume SP"=0.0, "MM PV"=0.0, "Start"=FALSE, "Home"=FALSE} ("PVT"), Variant=w405) -> (data=w403:T1, error out=w406:errorcluster)
            n196 = Unbundle By Name(w403) -> ("Mode"=w402:u16)
            n197 = case shown="1" w402 {
              tunnel: [u32 6618880 u32 14352335 u32 16775840 u32 16775840] -> w401
              tunnel: [u32 6618880 u32 16775840 u32 14352335 u32 16775840] -> w400
              tunnel: [u32 6618880 u32 16775840 u32 16775840 u32 14352335] -> w399
              frame 0, Default {
              }
              frame 1 {
              }
              frame 2 {
              }
              frame 3 {
              }
            }
            n198 = property on="Volume SP" class="DigNum (strict)"("NumText.BGColor"=w399) -> (error out=w396:errorcluster)  [unwired: 2 in, 1 out]
            n199 = property on="Flow SP" class="DigNum (strict)"("NumText.BGColor"=w400) -> (error out=w397:errorcluster)  [unwired: 2 in, 1 out]
            n200 = property on="Pressure SP" class="DigNum (strict)"("NumText.BGColor"=w401) -> (error out=w398:errorcluster)  [unwired: 2 in, 1 out]
            n201 = Merge Errors(w398, w397, w396, w406) -> (w409:errorcluster)
          }
          frame "Update UIP" {
            # "Duplicate this frame when creating new messages.  Change this comment in the duplicated frame to describe this message."
            n202 = Variant To Data(error in=w433, type=T1 {"Mode"=1, "Pressure PV"=0.0, "Pressure SP"=0.0, "Flow PV"=0.0, "Flow SP"=0.0, "Volume PV"=0.0, "Volume SP"=0.0, "MM PV"=0.0, "Start"=FALSE, "Home"=FALSE} ("PVT"), Variant=w431) -> (data=w429:T1, error out=w432:errorcluster)
            n203 = Unbundle By Name(w429) -> ("Mode"=w428:u16)
            n204 = case shown="1" w428 {
              tunnel: [u32 6618880 u32 14352335 u32 16775840 u32 16775840] -> w427
              tunnel: [u32 6618880 u32 16775840 u32 14352335 u32 16775840] -> w424
              tunnel: [u32 6618880 u32 16775840 u32 16775840 u32 14352335] -> w422
              frame 0, Default {
              }
              frame 1 {
              }
              frame 2 {
              }
              frame 3 {
              }
            }
            n205 = property on="Volume SP" class="DigNum (strict)"("NumText.BGColor"=w422) -> (error out=w423:errorcluster)  [unwired: 2 in, 1 out]
            n206 = property on="Flow SP" class="DigNum (strict)"("NumText.BGColor"=w424) -> (error out=w425:errorcluster)  [unwired: 2 in, 1 out]
            n207 = property on="Pressure SP" class="DigNum (strict)"("NumText.BGColor"=w427) -> (error out=w426:errorcluster)  [unwired: 2 in, 1 out]
            n208 = Merge Errors(w426, w425, w423, w432) -> (w435:errorcluster)
          }
          frame "Update UI Rotate" {
            # "Duplicate this frame when creating new messages.  Change this comment in the duplicated frame to describe this message."
            n209 = Variant To Data(error in=w455, type=T2 {"Mode"=1, "PV Angle"=0.0, "SP_Angle"=0.0, "Rotate Angle"=0.0, "Timeout"=0.0, "Start"=FALSE, "Home"=FALSE} ("Rotate"), Variant=w453) -> (data=w452:T2, error out=w454:errorcluster)
            n210 = Unbundle By Name(w452) -> ("Mode"=w451:u16)
            n211 = case shown="2" w451 {
              tunnel: [w458 w459] -> w450
              tunnel: [w458 w459] -> w449
              frame 1, Default {
                w458 = FALSE ("Visible")
              }
              frame 2 {
                w459 = TRUE ("Visible")
              }
            }
            n212 = property on="Rotate Angle" class="DigNum (strict)"("Visible"=w450) -> ()  [unwired: 2 in, 2 out]
            n213 = property on="Timeout" class="DigNum (strict)"("Visible"=w449) -> ()  [unwired: 2 in, 2 out]
            n214 = Merge Errors(w454) -> (w457:errorcluster)
          }
          frame "Load param" {
            w484 = T27 {"Q mix"=0.0, "Angle"=0.0, "KP"=750.0, "TN"=12.0, "PVT"={"Mode"=1, "Pressure PV"=0.0, "Pressure SP"=0.0, "Flow PV"=0.0, "Flow SP"=0.0, "Volume PV"=0.0, "Volume SP"=0.0, "MM PV"=0.0, "Start"=FALSE, "Home"=FALSE}, "Rotate"={"Mode"=1, "PV Angle"=0.0, "SP_Angle"=0.0, "Rotate Angle"=0.0, "Timeout"=0.0, "Start"=FALSE, "Home"=FALSE}, "Насос"={"Mode"=1, "Pressure PV"=0.0, "Pressure SP"=0.0, "Flow PV"=0.0, "Flow SP"=0.0, "Volume PV"=0.0, "Volume SP"=0.0, "MM PV"=0.0, "Start"=FALSE, "Home"=FALSE}, "KP 2"=750.0, "TN 2"=12.0} ("Save param")
            # "Duplicate this frame when creating new messages.  Change this comment in the duplicated frame to describe this message."
            n215 = call <vilib>:"Application Directory.vi"() -> ("Application Directory"=w490:path)
            n216 = Build Path(base path=w490, name or relative path="data\\drive.cfg" ("string")) -> (appended path=w488:path)
            n217 = call <vilib>:"Open Config Data.vi"("configuration file path"=w488) -> ("refnum"=w483:T31)  [unwired: 8 in, 2 out]
            n218 = call <userlib>:"Read INI Cluster__ogtk.vi"("INI Fomatted Cluster Type"=w484, "refnum"=w483) -> ("error out"=w487:errorcluster, "INI Fomatted Cluster"=w486:variant)  [unwired: 5 in, 3 out]
            n219 = Variant To Data(error in=w487, type=w484, Variant=w486) -> (data=w482:T27, error out=w485:errorcluster)
            n220 = Unbundle By Name(w482) -> ("Rotate"=w473:T2, "Q mix"=w479:dbl, "KP"=w478:sgl, "TN"=w477:sgl, "PVT"=w481:T1, "Насос"=w464:T1, "KP 2"=w462:sgl, "TN 2"=w461:sgl)  [unwired: 1 out]
            n221 = Bundle By Name(cluster=w473, "Start"=FALSE) -> (w460:T2)
            n222 = Bundle By Name(cluster=w481, "Start"=FALSE) -> (w474:T1)
            n223 = Bundle By Name(cluster=w464, "Start"=FALSE) -> (w463:T1)
            n224 = local write "TN 2"(w461) -> ()
            n225 = local write "KP 2"(w462) -> ()
            n226 = property on="Q" class="DigNum (strict)"("Value"=w479) -> ()  [unwired: 2 in, 2 out]
            n227 = local write "Rotate"(w460) -> ()
            n228 = local write "TN"(w477) -> ()
            n229 = local write "KP"(w478) -> ()
            n230 = local write "PVT"(w474) -> ()
            n231 = local write "Насос"(w463) -> ()
            n232 = call-poly <vilib>:"Delacor_lib_QMH_Enqueue Message (poly).vi"("Message Data"=w474, "Message"="Update UI", "Message Queue in"=w475) -> ("error out"=w471:errorcluster, "Message Queue out"=w470:refnum<class "Delacor_lib_QMH_Message Queue.lvclass">)  [unwired: 7 in]
            n233 = call-poly <vilib>:"Delacor_lib_QMH_Enqueue Message (poly).vi"("error in"=w471, "Message Data"=w460, "Message"="Update UI Rotate", "Message Queue in"=w470) -> ("Message Queue out"=w467:refnum<class "Delacor_lib_QMH_Message Queue.lvclass">)  [unwired: 6 in, 1 out]
            n234 = call-poly <vilib>:"Delacor_lib_QMH_Enqueue Message (poly).vi"("Message Data"=w463, "Message"="Update UIP", "Message Queue in"=w467) -> ("error out"=w468:errorcluster)  [unwired: 7 in, 1 out]
            n235 = Merge Errors(w468, w485, w493) -> (w492:errorcluster)
          }
          frame "Setts" {
            # "Duplicate this frame when creating new messages.  Change this comment in the duplicated frame to describe this message."
            n236 = Variant To Data(error in=w506, type=T15 {"Vm0"=8.0, "aa"=8.0, "bb"=8.0, "K0"=8.0, "A"=8.0, "B"=8.0} ("Расчёты"), Variant=w505) -> (data=w494:T15, error out=w502:errorcluster)
            n237 = Unbundle By Name(w494) -> ("Vm0"=w501:dbl, "aa"=w500:dbl, "bb"=w499:dbl, "K0"=w497:dbl, "A"=w498:dbl, "B"=w496:dbl)
            n238 = Bundle By Name(cluster=w507, "Расчёты"=w494) -> (w503:T10)
            n239 = call "Set PVT Volume Param.vi"("B"=w496, "A"=w498, "K0"=w497, "b"=w499, "a"=w500, "Vm0"=w501) -> ("error out"=w495:errorcluster)  [unwired: 4 in, 1 out]
            n240 = Merge Errors(w495, w502) -> (w508:errorcluster)
          }
          frame "Read Setts" {
            # "Duplicate this frame when creating new messages.  Change this comment in the duplicated frame to describe this message."
            n241 = call "Get Settings.vi"("wait for reply (T)"=TRUE) -> ("error out"=w517:errorcluster, "Main"=w518:T30)  [unwired: 8 in, 1 out]
            n242 = Unbundle By Name(w518) -> ("Расчёты"=w516:T15)
            n243 = Unbundle By Name(w516) -> ("Vm0"=w515:dbl, "aa"=w514:dbl, "bb"=w513:dbl, "K0"=w511:dbl, "A"=w512:dbl, "B"=w510:dbl)
            n244 = Bundle By Name(cluster=w521, "Расчёты"=w516) -> (w520:T10)
            n245 = call "Set PVT Volume Param.vi"("B"=w510, "A"=w512, "K0"=w511, "b"=w513, "a"=w514, "Vm0"=w515) -> ("error out"=w509:errorcluster)  [unwired: 4 in, 1 out]
            n246 = Merge Errors(w509, w517) -> (w522:errorcluster)
          }
          frame "Temp Data" {
            # "Duplicate this frame when creating new messages.  Change this comment in the duplicated frame to describe this message."
            n247 = Variant To Data(error in=w528, type=dbl[] [] ("Temp array"), Variant=w527) -> (data=w523:dbl[], error out=w525:errorcluster)
            n248 = Bundle By Name(cluster=w529, "Temp array"=w523) -> (w524:T10)
            n249 = Merge Errors(w525) -> (w530:errorcluster)
          }
          frame "PLC Read" {
            # "Duplicate this frame when creating new messages.  Change this comment in the duplicated frame to describe this message."
            n250 = Unbundle By Name(w532) -> ("MB"=w555:refnum<class "Modbus Master.lvclass">)
            n251 = Unbundle By Name(w532) -> ("Temp array"=w545:dbl[])
            n252 = call-dynamic "Read Holding Registers.vi"("number of inputs"=u16 15, "starting address"=u16 0, "Modbus master in"=w555) -> ("error out"=w551:errorcluster, "register values"=w549:u16[], "Modbus master out"=w550:refnum<class "Modbus Master.lvclass">)  [unwired: 6 in]
            n253 = local read "PVT"() -> (w548:T1)
            n254 = property on="Q" class="DigNum (strict)"() -> ("Value"=w542:dbl)  [unwired: 2 in, 2 out]
            n255 = call "PLC Unpuck.vi"("PVT in"=w548, "register values"=w549) -> ("PVT"=w533:T1)  [unwired: 9 in]
            n256 = Bundle By Name(cluster=w532, "MB"=w550) -> (w539:T10)
            n257 = Index Array(array=w545) -> (element=w544:dbl)  [unwired: 1 in]
            n258 = Unbundle By Name(w533) -> ("Pressure PV"=w535:dbl)
            "P" <- w535
            n259 = local write "PVT"(w533) -> ()
            n260 = call "Set Output.vi"("Value %"=w535, "Channel"=u16 3, "Module ID"=-1) -> ("error out"=w534:errorcluster)  [unwired: 8 in]
            n261 = Unbundle By Name(w532) -> ("Расчёты"=w531:T15)
            n262 = case shown="No Error" w551 {
              tunnel: [w567 w596] -> w552
              tunnel: T25 {"Pressure PV"=0.0, "Flow PV"=0.0, "Volume PV"=0.0, "Position_MM"=0.0, "Volume corrected"=0.0, "mix rpm"=0.0} ("Pump_data") -> [w594 _]
              tunnel: [w592 _] -> w546
              tunnel: w533 -> [w591 _]
              tunnel: w544 -> [w589 _]
              tunnel: [w587 _] -> w543
              tunnel: w542 -> [w581 _]
              tunnel: [w580 _] -> w541
              tunnel: w540 -> [w568 _]
              tunnel: w539 -> [_ w599]
              tunnel: [w565 _] -> w538
              tunnel: w531 -> [w558 _]
              frame No Error {
                w571 = T26."Disabled and Grayed Out" ("f")
                w570 = T26."Enabled" ("Disabled")
                n263 = property on="on" class="Bool (strict)"() -> ("Value"=w585:bool)  [unwired: 2 in, 2 out]
                n264 = Unbundle By Name(w591) -> ("Start"=w569:bool, "Pressure PV"=w575:dbl, "Flow PV"=w564:dbl, "Volume PV"=w590:dbl, "MM PV"=w583:dbl)
                n265 = local read "P3"() -> (w561:dbl)
                n266 = local read "P2"() -> (w562:dbl)
                n267 = Less?(x=w583, y=4.0) -> (x < y?=w586:bool)
                n268 = Subtract(x=w562, y=w561) -> (x-y=w560:dbl)
                n269 = call "Corrected Volume PVT.vi"("Расчёты"=w558, "h"=w583, "T"=w589, "P"=w575) -> ("error out"=w587:errorcluster, "Vcorr"=w588:dbl)  [unwired: 6 in]
                n270 = And(x=w586, y=w585) -> (x .and. y?=w582:bool)
                n271 = call-poly <vilib>:"Delacor_lib_QMH_Enqueue Message (poly).vi"("Message"="PLCP Read", "Message Queue in"=w568) -> ("error out"=w567:errorcluster)  [unwired: 8 in, 1 out]
                n272 = Greater Or Equal?(x=0.25, y=w575) -> (x >= y?=w573:bool)
                n273 = Absolute Value(x=w560) -> (abs(x)=w559:dbl)
                n274 = Bundle By Name(cluster=w594, "Pressure PV"=w575, "Flow PV"=w564, "Volume PV"=w590, "Position_MM"=w583, "Volume corrected"=w588, "mix rpm"=w581) -> (w593:T25)
                n275 = Build Array(w564) -> (w563:dbl[])
                n276 = case shown="True" w582 {
                  frame False {
                  }
                  frame True {
                    n277 = property on="on" class="Bool (strict)"("Val(Sgnl)"=FALSE ("Value (Signaling)")) -> ()  [unwired: 2 in, 2 out]
                  }
                }
                n278 = Select(t=i32[] [] ("Disabled Items []"), s=w573, f=i32[] [3] ("Disabled Items []")) -> (s? t:f=w577:i32[])
                n279 = property on="Mode" class="Ring (strict)"("Disabled Items []"=w577) -> (error out=w580:errorcluster)  [unwired: 2 in, 1 out]
                n280 = Select(t=w571, s=w569, f=w570) -> (s? t:f=w572:T26)
                n281 = Select(t=w570, s=w573, f=w571) -> (s? t:f=w574:T26)
                n282 = call "New data.vi"("dP"=w559, "Q"=w563) -> ("error out"=w565:errorcluster)  [unwired: 9 in]
                n283 = property on="Mode" class="Ring (strict)"("DisabledEnum"=w572) -> ()  [unwired: 2 in, 2 out]
                n284 = property on="Home" class="Bool (strict)"("DisabledEnum"=w574) -> ()  [unwired: 2 in, 2 out]
                n285 = call "Pump_Data.vi"("Pump_data"=w593) -> ("error out"=w592:errorcluster)  [unwired: 10 in]
              }
              frame Error {
                n286 = Unbundle By Name(w599) -> ("Plan Enqueuer"=w598:refnum<class "Message Enqueuer.lvclass">)
                n287 = call <vilib>:"Add Event.vi"("Action"="PLC Connect", "Plan Enqueuer"=w598) -> ("error out"=w596:errorcluster)  [unwired: 7 in, 2 out]
              }
            }
            n288 = Merge Errors(w538, w541, w543, w546, w552, w551, w557, w534) -> (w556:errorcluster)
          }
          frame "PLCP Read" {
            # "Duplicate this frame when creating new messages.  Change this comment in the duplicated frame to describe this message."
            n289 = Unbundle By Name(w605) -> ("MB"=w612:refnum<class "Modbus Master.lvclass">)
            n290 = call-dynamic "Read Holding Registers.vi"("number of inputs"=u16 15, "starting address"=u16 34, "Modbus master in"=w612) -> ("error out"=w608:errorcluster, "register values"=w606:u16[], "Modbus master out"=w607:refnum<class "Modbus Master.lvclass">)  [unwired: 6 in]
            n291 = local read "Насос"() -> (w602:T1)
            n292 = call "PLC Unpuck.vi"("PVT in"=w602, "register values"=w606) -> ("PVT"=w601:T1)  [unwired: 9 in]
            n293 = Bundle By Name(cluster=w605, "MB"=w607) -> (w603:T10)
            n294 = local write "Насос"(w601) -> ()
            n295 = case shown="No Error" w608 {
              tunnel: [w631 w636] -> w609
              tunnel: w601 -> [w626 _]
              tunnel: w604 -> [_ _]
              tunnel: w603 -> [w632 w639]
              tunnel: [w617 _] -> w600
              frame No Error {
                n296 = Unbundle By Name(w632) -> ("Plan Enqueuer"=w630:refnum<class "Message Enqueuer.lvclass">)
                n297 = Unbundle By Name(w626) -> ("Pressure PV"=w621:dbl, "Flow PV"=w620:dbl, "Volume PV"=w615:dbl)
                "Pressure PV 2" <- w621
                "MM PV" <- w615
                n298 = Unbundle By Name(w626) -> ("Start"=w633:bool, "MM PV"=→"Pressure PV":dbl)
                n299 = local read "P3"() -> (w618:dbl)
                n300 = local read "P2"() -> (w619:dbl)
                n301 = Less?(x=w621, y=0.25) -> (x < y?=w622:bool)
                n302 = call <vilib>:"Add Event.vi"("Action"="PLC Read", "Plan Enqueuer"=w630) -> ("error out"=w631:errorcluster)  [unwired: 7 in, 2 out]
                n303 = call "Pump2 data.vi"("P3"=w618, "P2"=w619, "Volume PV"=w615, "Flow PV"=w620, "Pressure PV"=w621) -> ("error out"=w617:errorcluster)  [unwired: 6 in]
                n304 = Select(t=T26."Disabled and Grayed Out" ("f"), s=w633, f=T26."Enabled" ("Disabled")) -> (s? t:f=w628:T26)
                n305 = property on="Mode" class="Ring (strict)"("DisabledEnum"=w628) -> ()  [unwired: 2 in, 2 out]
                n306 = Select(t=T26."Enabled" ("Disabled"), s=w622, f=T26."Disabled and Grayed Out") -> (s? t:f=w616:T26)
                n307 = property on="Home" class="Bool (strict)"("DisabledEnum"=w616) -> ()  [unwired: 2 in, 2 out]
              }
              frame Error {
                n308 = Unbundle By Name(w639) -> ("Plan Enqueuer"=w638:refnum<class "Message Enqueuer.lvclass">)
                n309 = call <vilib>:"Add Event.vi"("Action"="PLC Connect", "Plan Enqueuer"=w638) -> ("error out"=w636:errorcluster)  [unwired: 7 in, 2 out]
              }
            }
            n310 = Merge Errors(w600, w609, w608, w614) -> (w613:errorcluster)
          }
          frame "PLC Connect" {
            # "Duplicate this frame when creating new messages.  Change this comment in the duplicated frame to describe this message."
            n311 = call-poly <vilib>:"Create Modbus Instance.vi"("connect timeout ms"=1000, "address"="192.168.0.200") -> ("error out"=w645:errorcluster, "TCP master instance"=w646:refnum<class "Modbus Master.lvclass">)  [unwired: 8 in]
            n312 = Unbundle By Name(w644) -> ("Plan Enqueuer"=w643:refnum<class "Message Enqueuer.lvclass">)
            n313 = case shown="No Error" w645 {
              tunnel: w643 -> [w656 w662]
              tunnel: [w658 w661] -> w642
              tunnel: [w653 _] -> w641
              tunnel: w640 -> [w659 _]
              frame No Error {
                n314 = call <vilib>:"Add Event.vi"("Action"="PLC Read", "Plan Enqueuer"=w656) -> ("error out"=w658:errorcluster)  [unwired: 7 in, 2 out]
                n315 = call-poly <vilib>:"Delacor_lib_QMH_Enqueue Message (poly).vi"("Message"="Write PID", "Message Queue in"=w659) -> ("error out"=w654:errorcluster, "Message Queue out"=w655:refnum<class "Delacor_lib_QMH_Message Queue.lvclass">)  [unwired: 8 in]
                n316 = call-poly <vilib>:"Delacor_lib_QMH_Enqueue Message (poly).vi"("error in"=w654, "Message"="ReadDO", "Message Queue in"=w655) -> ("error out"=w653:errorcluster)  [unwired: 7 in, 1 out]
              }
              frame Error {
                n317 = call <vilib>:"Add Event.vi"("Action"="PLC Connect", "Plan Enqueuer"=w662) -> ("error out"=w661:errorcluster)  [unwired: 7 in, 2 out]
              }
            }
            n318 = Bundle By Name(cluster=w644, "MB"=w646) -> (w647:T10)
            n319 = Merge Errors(w641, w642, w645, w651) -> (w650:errorcluster)
          }
          frame "Mix" {
            # "Duplicate this frame when creating new messages.  Change this comment in the duplicated frame to describe this message."
            n320 = Variant To Data(error in=w678, type="MIX", Variant=w677) -> (data=w674:T3, error out=w675:errorcluster)
            n321 = Unbundle By Name(w674) -> ("Q"=w672:dbl, "on"=w673:bool)
            n322 = Multiply(x=0.03333333333333333, y=w672) -> (x*y=w665:dbl)
            n323 = Select(t=w665, s=w673, f=0.0) -> (s? t:f=w666:dbl)
            n324 = call "Set Output.vi"("Value %"=w666, "Channel"=u16 2, "Module ID"=-1) -> ("error out"=w669:errorcluster)  [unwired: 8 in]
            n325 = Merge Errors(w669, w675) -> (w679:errorcluster)
          }
          frame "PLC Send" {
            # "Duplicate this frame when creating new messages.  Change this comment in the duplicated frame to describe this message."
            n326 = Variant To Data(error in=w694, type="PVT", Variant=w693) -> (data=w680:T1, error out=w692:errorcluster)
            n327 = Unbundle By Name(w690) -> ("MB"=w689:refnum<class "Modbus Master.lvclass">)
            n328 = call "PLC Puck.vi"("PVT"=w680) -> ("appended array"=w687:u16[])  [unwired: 10 in]
            n329 = call-dynamic "Write Multiple Holding Registers.vi"("registers to write"=w687, "starting address"=u16 16, "Modbus master in"=w689) -> ("error out"=w686:errorcluster, "Modbus master out"=w684:refnum<class "Modbus Master.lvclass">)  [unwired: 7 in]
            n330 = Bundle By Name(cluster=w690, "MB"=w684) -> (w685:T10)
            n331 = call-poly <vilib>:"Delacor_lib_QMH_Enqueue Message (poly).vi"("Message Data"=w680, "Message"="Update UI", "Message Queue in"=w682) -> ("error out"=w683:errorcluster)  [unwired: 7 in, 1 out]
            n332 = Merge Errors(w683, w686, w692) -> (w695:errorcluster)
          }
          frame "PLCP Send" {
            w696 = FALSE ("element")
            # "Duplicate this frame when creating new messages.  Change this comment in the duplicated frame to describe this message."
            n333 = Variant To Data(error in=w724, type="Насос", Variant=w723) -> (data=w711:T1, error out=w722:errorcluster)
            n334 = Unbundle By Name(w721) -> ("MB"=w720:refnum<class "Modbus Master.lvclass">)
            n335 = call "PLC Puck.vi"("PVT"=w711) -> ("appended array"=w718:u16[])  [unwired: 10 in]
            n336 = Build Array(w696, w696, w696, w696, w696, w696, w696, w696, "K 1", "K 2", "K 3", "K 4", "K 5", "K 6", "KE", "КМ20-40М") -> (w699:bool[])
            n337 = Boolean Array To Number(Boolean array=w699) -> (number=w698:u32)
            n338 = To Unsigned Word Integer(number=w698) -> (unsigned 16bit integer=w697:u16)
            n339 = Replace Array Subset(array=w718, new element=w697, index=0) -> (w709:u16[])
            n340 = call-dynamic "Write Multiple Holding Registers.vi"("registers to write"=w709, "starting address"=u16 50, "Modbus master in"=w720) -> ("error out"=w717:errorcluster, "Modbus master out"=w715:refnum<class "Modbus Master.lvclass">)  [unwired: 7 in]
            n341 = Bundle By Name(cluster=w721, "MB"=w715) -> (w716:T10)
            n342 = call-poly <vilib>:"Delacor_lib_QMH_Enqueue Message (poly).vi"("Message Data"=w711, "Message"="Update UIP", "Message Queue in"=w713) -> ("error out"=w714:errorcluster)  [unwired: 7 in, 1 out]
            n343 = Merge Errors(w714, w717, w722) -> (w725:errorcluster)
          }
          frame "PLC Send Rotate" {
            # "Duplicate this frame when creating new messages.  Change this comment in the duplicated frame to describe this message."
            n344 = Variant To Data(error in=w744, type="Rotate", Variant=w743) -> (data=w730:T2, error out=w742:errorcluster)
            n345 = Unbundle By Name(w734) -> ("Rotate_ID"=w733:i32)
            n346 = Unbundle By Name(w730) -> ("Start"=w726:bool, "SP_Angle"=w735:dbl)
            n347 = Multiply(x=w735, y=18204.444444444445) -> (x*y=w732:dbl)
            n348 = call "Set_Position.vi"("Position"=w732, "Module ID"=w733) -> ("error out"=w737:errorcluster)  [unwired: 9 in]
            n349 = Select(t=50.0 ("Speed"), s=w726, f=0.0) -> (s? t:f=w729:dbl)
            n350 = call "Set_Speed.vi"("error in"=w737, "Speed"=w729, "Module ID"=w733) -> ("error out"=w738:errorcluster)  [unwired: 8 in]
            n351 = call-poly <vilib>:"Delacor_lib_QMH_Enqueue Message (poly).vi"("Message Data"=w730, "Message"="Update UI Rotate", "Message Queue in"=w740) -> ("error out"=w741:errorcluster)  [unwired: 7 in, 1 out]
            n352 = Merge Errors(w738, w741, w742) -> (w745:errorcluster)
          }
          frame "Write PID" {
            # "Duplicate this frame when creating new messages.  Change this comment in the duplicated frame to describe this message."
            n353 = Unbundle By Name(w758) -> ("MB"=w757:refnum<class "Modbus Master.lvclass">)
            n354 = call "Float_TO_WORD.vi"("FLOAT"="TN") -> ("second_Word"=w747:u16, "first_Word"=w748:u16)  [unwired: 9 in]
            n355 = call "Float_TO_WORD.vi"("FLOAT"="KP") -> ("second_Word"=w749:u16, "first_Word"=w750:u16)  [unwired: 9 in]
            n356 = Build Array(w750, w749, w748, w747) -> (w746:u16[])
            n357 = call-dynamic "Write Multiple Holding Registers.vi"("registers to write"=w746, "starting address"=u16 28, "Modbus master in"=w757) -> ("error out"=w755:errorcluster, "Modbus master out"=w753:refnum<class "Modbus Master.lvclass">)  [unwired: 7 in]
            n358 = Bundle By Name(cluster=w758, "MB"=w753) -> (w754:T10)
            n359 = Merge Errors(w755) -> (w759:errorcluster)
          }
          frame "Write PIDP" {
            # "Duplicate this frame when creating new messages.  Change this comment in the duplicated frame to describe this message."
            n360 = Unbundle By Name(w772) -> ("MB"=w771:refnum<class "Modbus Master.lvclass">)
            n361 = call "Float_TO_WORD.vi"("FLOAT"="TN 2") -> ("second_Word"=w763:u16, "first_Word"=w764:u16)  [unwired: 9 in]
            n362 = call "Float_TO_WORD.vi"("FLOAT"="KP 2") -> ("second_Word"=w765:u16, "first_Word"=w766:u16)  [unwired: 9 in]
            n363 = Build Array(w766, w765, w764, w763) -> (w762:u16[])
            n364 = call-dynamic "Write Multiple Holding Registers.vi"("registers to write"=w762, "starting address"=u16 62, "Modbus master in"=w771) -> ("error out"=w769:errorcluster, "Modbus master out"=w767:refnum<class "Modbus Master.lvclass">)  [unwired: 7 in]
            n365 = Bundle By Name(cluster=w772, "MB"=w767) -> (w768:T10)
            n366 = Merge Errors(w769) -> (w773:errorcluster)
          }
          frame "PLC Home" {
            # "Duplicate this frame when creating new messages.  Change this comment in the duplicated frame to describe this message."
            n367 = Unbundle By Name(w782) -> ("MB"=w781:refnum<class "Modbus Master.lvclass">)
            n368 = Build Array(u16 1 ("starting address")) -> (w774:u16[])
            n369 = call-dynamic "Write Multiple Holding Registers.vi"("registers to write"=w774, "starting address"=u16 16, "Modbus master in"=w781) -> ("error out"=w780:errorcluster, "Modbus master out"=w778:refnum<class "Modbus Master.lvclass">)  [unwired: 7 in]
            n370 = Bundle By Name(cluster=w782, "MB"=w778) -> (w779:T10)
            n371 = Merge Errors(w780, w777) -> (w783:errorcluster)
          }
          frame "PLCP Home" {
            w794 = u16 50 ("starting address")
            # "Duplicate this frame when creating new messages.  Change this comment in the duplicated frame to describe this message."
            n372 = Unbundle By Name(w802) -> ("MB"=w797:refnum<class "Modbus Master.lvclass">)
            n373 = call-dynamic "Read Holding Registers.vi"("number of inputs"=u16 1, "starting address"=w794, "Modbus master in"=w797) -> ("error out"=w795:errorcluster, "register values"=w791:u16[], "Modbus master out"=w796:refnum<class "Modbus Master.lvclass">)  [unwired: 6 in]
            n374 = Index Array(array=w791) -> (element=w790:u16)  [unwired: 1 in]
            n375 = Number To Boolean Array(number=w790) -> (Boolean array=w789:bool[])
            n376 = Replace Array Subset(array=w789, new element=TRUE, index=0) -> (w785:bool[])
            n377 = Boolean Array To Number(Boolean array=w785) -> (number=w784:u32)
            n378 = Replace Array Subset(array=w791, new element=w784, index=0) -> (w792:u16[])
            n379 = call-dynamic "Write Multiple Holding Registers.vi"("error in"=w795, "registers to write"=w792, "starting address"=w794, "Modbus master in"=w796) -> ("error out"=w801:errorcluster, "Modbus master out"=w799:refnum<class "Modbus Master.lvclass">)  [unwired: 6 in]
            n380 = Bundle By Name(cluster=w802, "MB"=w799) -> (w800:T10)
            n381 = Merge Errors(w801, w798) -> (w803:errorcluster)
          }
          frame "PLC Rotate Home" {
            # "Duplicate this frame when creating new messages.  Change this comment in the duplicated frame to describe this message."
            n382 = Unbundle By Name(w807) -> ("Rotate_ID"=w805:i32)
            n383 = call "Go_Home.vi"("Module ID"=w805) -> ("error out"=w804:errorcluster)  [unwired: 10 in]
            n384 = Merge Errors(w804, w806) -> (w808:errorcluster)
          }
          frame "Kinco Status" {
            # "Duplicate this frame when creating new messages.  Change this comment in the duplicated frame to describe this message."
            n385 = Variant To Data(error in=w821, type=T11 {"Module ID"=-1, "Connection"=FALSE, "is Home?"=FALSE, "Position"=0.0, "Done?"=FALSE} ("Drive_Status Argument"), Variant=w820) -> (data=w812:T11, error out=w819:errorcluster)
            n386 = Unbundle By Name(w812) -> ("Module ID"=w815:i32)
            n387 = Unbundle By Name(w818) -> ("Rotate_ID"=w814:i32)
            n388 = Equal?(x=w814, y=w815) -> (x = y?=w813:bool)
            n389 = case shown="True" w813 {
              tunnel: w818 -> [w823 w833]
              tunnel: [w823 w832] -> w816
              tunnel: w812 -> [_ w827]
              tunnel: [_ w828] -> w811
              tunnel: w810 -> [_ w825]
              tunnel: [_ w824] -> w809
              frame False {
              }
              frame True {
                n390 = Unbundle By Name(w827) -> ("Done?"=w831:bool)
                n391 = Bundle By Name(cluster=w833, "Rotate status"=w827) -> (w832:T10)
                n392 = call <vilib>:"Boolean Crossing PtByPt.vi"("direction"=enum16{"either", "false-true", "true-false"}."false-true", "input"=w831) -> ("crossing"=w829:bool)  [unwired: 1 in]
                n393 = case shown="True" w829 {
                  tunnel: [_ w836] -> w828
                  tunnel: w825 -> [_ w835]
                  frame False {
                  }
                  frame True {
                    n394 = call-poly <vilib>:"Delacor_lib_QMH_Enqueue Message (poly).vi"("Message"="RStop", "Message Queue in"=w835) -> ("error out"=w836:errorcluster)  [unwired: 8 in, 1 out]
                  }
                }
                n395 = call-poly <vilib>:"Delacor_lib_QMH_Enqueue Message (poly).vi"("Message"="PLC Read Rotate", "Message Queue in"=w825) -> ("error out"=w824:errorcluster)  [unwired: 8 in, 1 out]
              }
            }
            n396 = Merge Errors(w809, w811, w819) -> (w822:errorcluster)
          }
          frame "---Exit and Error Handling---" {
            # "Separator - The following cases handle errors and exit messages."
          }
          frame "Simulate MHL Error" {
            # "#DQMH_HowTo The 'Simulate MHL Error' button  illustrates how the MHL handles errors. This event is instructional in nature and can be removed."
            # "Simulate an error occurring at the MHL"
            n397 = call "Module Name--constant.vi"() -> ("Module Name"=w839:string)  [unwired: 11 in]
            n398 = xnode "Error Ring"("parameter 0"=w839) -> ("error out"=w841:errorcluster)
            n399 = Merge Errors(w843, w841) -> (w842:errorcluster)
          }
          frame "Error" {
            # "#CodeRecommended - If you ever change the name of this \"Error\" message, you'll need to update the name in the Check Loop Error.vi as well."
            # "#CodeRecommended - If the module is running in standalone mode (External Launch = FALSE), this code will pop up an error dialog and call the 'Exit' message if an error occurs. Add more fine-grained error handling here."
            # "Error - Check the error message data and respond accordingly. This message is sent by the \"Error Handler\" VIs at the end of each loop in this application."
            n400 = property class="Module Admin"(reference=w852) -> ("Accessors:External Launch"=w851:bool)  [unwired: 1 in, 2 out]
            n401 = Variant To Data(error in=w860, type=errorcluster {"status"=FALSE, "code"=0, "source"=""} ("error constant"), Variant=w854) -> (data=w861:errorcluster, error out=w858:errorcluster)
            n402 = call "Error Reported.vi"("Error"=w861) -> ()  [unwired: 10 in, 1 out]
            n403 = case shown="False" w851 {
              tunnel: [w866 _] -> w857
              tunnel: w853 -> [w864 _]
              tunnel: w861 -> [w865 _]
              frame False {
                # "If the module is running standalone, then pop up an error dialog and call the \"Exit\" message."
                n404 = call <vilib>:"Simple Error Handler.vi"("error in (no error)"=w865) -> ()  [unwired: 4 in, 5 out]
                n405 = call-poly <vilib>:"Delacor_lib_QMH_Enqueue Message (poly).vi"("Priority Message? (F)"=TRUE, "Message"="Exit", "Message Queue in"=w864) -> ("error out"=w866:errorcluster)  [unwired: 7 in, 1 out]
              }
              frame True {
                # "If the module was launched externally, calling the Error Reported broadcast VI is the only action performed by the \"Error\" message. The module's caller can then process the error appropriately."
              }
            }
            n406 = Merge Errors(w858, w857) -> (w856:errorcluster)
            n407 = local write "error out"(w856) -> ()
          }
          frame "Exit" {
            w900 = 91  # 91: not all Exit messages will have an argument
            w902 = TRUE  # Stop the VI
            # "Release the message queue reference"
            # "Exit - Exit the application."
            n408 = Variant To Data(error in=w909, type=T17 {"Origin"="", "Exit via Stop Module Req?"=FALSE, "Wait for Module to stop?"=FALSE} ("Stop Argument"), Variant=w901) -> (data=w898:T17, error out=w905:errorcluster)
            n409 = Unbundle By Name(w890) -> ("MB"=w889:refnum<class "Modbus Master.lvclass">, "Plan Enqueuer"=w872:refnum<class "Message Enqueuer.lvclass">)
            n410 = call <vilib>:"Clear Errors.vi"("error in (no error)"=w905, "specific error code to clear (0: all)"=w900) -> ("error out"=w908:errorcluster)  [unwired: 4 in, 1 out]
            n411 = call <vilib>:"Application Directory.vi"() -> ("Application Directory"=w887:path)
            n412 = control-ref of="This VI"() -> (w897:refnum<vi>)
            n413 = Build Path(base path=w887, name or relative path="data\\drive.cfg" ("string")) -> (appended path=w885:path)
            n414 = call-dynamic "Shutdown.vi"("Modbus master in"=w889) -> ("error out"=w888:errorcluster)  [unwired: 10 in]
            n415 = call-dynamic "Delacor_lib_QMH_Release Message Queue.vi"("error in"=w908, "Message Queue"=w903) -> ("error out"=w907:errorcluster)  [unwired: 9 in]
            n416 = call <vilib>:"Stop.vi"("Plan Enqueuer"=w872) -> ("error out"=w870:errorcluster)  [unwired: 10 in]
            n417 = call "Handle Exit.vi"("Stop Argument"=w898, "Admin in"=w896, "VI reference"=w897) -> ("error out"=w904:errorcluster)  [unwired: 7 in, 1 out]
            n418 = call <vilib>:"Open Config Data.vi"("configuration file path"=w885) -> ("refnum"=w884:T31)  [unwired: 8 in, 2 out]
            n419 = call "Set_Speed.vi"("Speed"=0.0, "Module ID"=-1) -> ("error out"=w893:errorcluster)  [unwired: 9 in]
            n420 = Merge Errors(w888, w870) -> (w871:errorcluster)
            n421 = call "Stop Module.vi"("error in"=w893, "Module ID"=-1) -> ("error out"=w891:errorcluster)  [unwired: 9 in]
            n422 = local read "TN 2"() -> (w867:sgl)
            n423 = local read "Насос"() -> (w869:T1)
            n424 = local read "KP 2"() -> (w868:sgl)
            n425 = property on="Q" class="DigNum (strict)"() -> ("Value"=w878:dbl)  [unwired: 2 in, 2 out]
            n426 = local read "Rotate"() -> (w873:T2)
            n427 = local read "PVT"() -> (w875:T1)
            n428 = local read "TN"() -> (w876:sgl)
            n429 = local read "KP"() -> (w877:sgl)
            n430 = Bundle By Name(cluster=T27 {"Q mix"=0.0, "Angle"=0.0, "KP"=750.0, "TN"=12.0, "PVT"={"Mode"=1, "Pressure PV"=0.0, "Pressure SP"=0.0, "Flow PV"=0.0, "Flow SP"=0.0, "Volume PV"=0.0, "Volume SP"=0.0, "MM PV"=0.0, "Start"=FALSE, "Home"=FALSE}, "Rotate"={"Mode"=1, "PV Angle"=0.0, "SP_Angle"=0.0, "Rotate Angle"=0.0, "Timeout"=0.0, "Start"=FALSE, "Home"=FALSE}, "Насос"={"Mode"=1, "Pressure PV"=0.0, "Pressure SP"=0.0, "Flow PV"=0.0, "Flow SP"=0.0, "Volume PV"=0.0, "Volume SP"=0.0, "MM PV"=0.0, "Start"=FALSE, "Home"=FALSE}, "KP 2"=750.0, "TN 2"=12.0} ("Save param"), "Q mix"=w878, "Angle"=0.0, "KP"=w877, "TN"=w876, "PVT"=w875, "Rotate"=w873, "Насос"=w869, "KP 2"=w868, "TN 2"=w867) -> (w879:T27)
            n431 = call <userlib>:"Write INI Cluster__ogtk.vi"("INI Fomatted Cluster"=w879, "refnum"=w884) -> ("error out"=w883:errorcluster, "dup refnum"=w882:T31)  [unwired: 8 in]
            n432 = call <vilib>:"Close Config Data.vi"("error in (no error)"=w883, "refnum"=w882) -> ("error out"=w881:errorcluster)  [unwired: 8 in, 1 out]
            n433 = Merge Errors(w881, w871, w891, w907, w904) -> (w906:errorcluster)
          }
          frame Default {
            # "'Default' case only runs if there is a message that isn't defined in any of the other cases.  Output a programming error."
            n434 = call "Module Name--constant.vi"() -> ("Module Name"=w910:string)  [unwired: 11 in]
            n435 = xnode "Error Ring"("parameter 0"=w911, "parameter 1"=w910) -> ("error out"=w915:errorcluster)
            n436 = Merge Errors(w913, w915) -> (w914:errorcluster)
          }
        }
        n437 = call-dynamic "Delacor_lib_QMH_Error Handler - Message Handling Loop.vi"("error in"=w221, "Message Queue in"=w211) -> ("dup error in"=w218:errorcluster)  [unwired: 8 in, 1 out]
      }
    }
    frame Error {
      # "Synchronize Caller Events.vi will inform Start Module.vi that the module has launched and will let the code calling Start Module.vi register for broadcasts and would permit the caller receive the broadcast that an error occurred at launch time."
      n438 = call-dynamic "Delacor_lib_QMH_Release Message Queue.vi"("error in"=w926, "Message Queue"=w924) -> ("error out"=w925:errorcluster)  [unwired: 9 in]
      n439 = call "Synchronize Caller Events.vi"("Singleton Module Admin in"=w927) -> ("error out"=w932:errorcluster)  [unwired: 9 in, 1 out]
      n440 = call "Module Name--constant.vi"() -> ("Module Name"=w930:string)  [unwired: 11 in]
      n441 = Format Into String(format string="An error occurred during initialization. %s is no longer running.", w930) -> (resulting string=w928:string)  [unwired: 2 in, 1 out]
      n442 = Merge Errors(w925, w932) -> (w933:errorcluster)
      n443 = call "Error Reported.vi"("Additional Information"=w928, "Error"=w933) -> ()  [unwired: 9 in, 1 out]
    }
  }
  n444 = Merge Errors(w28, w31) -> (w27:errorcluster)
  n445 = call "Close Module.vi"("error in (no error)"=w27, "Module Admin in"=w23) -> ("error out"=w29:errorcluster, "External Launch"=w18:bool, "Module Admin out"=w19:refnum<class "Delacor_lib_QMH_Module Admin.lvclass">)  [unwired: 7 in]
  n446 = Unregister For Events(event registration refnum=w22, error in=w29) -> (error out=w26:errorcluster)
  "error out" <- w26
  n447 = case "External Launch?" shown="True" w18 {
    tunnel: w26 -> [_ _]
    frame False {
    }
    frame True {
      n448 = invoke class="VI" method="FP.Close"() -> ()  [unwired: 3 in, 3 out]
    }
  }
  n449 = local write "Module Admin"(w19) -> ()
